vi "映射处理_kc705.vi"() -> ()   [LabVIEW 2017]
uses:
  <vilib>/Utility/file.llb/Read Delimited Spreadsheet (string).vi
panel:
  in  "-N":bool=TRUE
  in  "prefix":string="HPC_"
  out "initialized array":string[][](array[string])
  out "all rows":string[][](array[string])=[["VO0", "LA02_P"], ["VO1", "HA06_P"], ["VO2", "HA10_P"], ["VO3", "HA15_P"], ["VO4", "LA20_P"], ["VO5", "HB02_P"], ["VO6", "HB00_P"], ["VO7", "LA24_P"], ["VO8", "HB13_P"], ["VO9", "HB16_P"], ["VO10", "LA01_P"], ["VO11", "HA08_P"], ["VO12", "HA12_P"], ["VO13", "HA20_P"], ["VO14", "LA19_P"], ["VO15", "LA23_P"], ["VO16", "HB04_P"], ["VO17", "HB08_P"], ["VO18", "HB15_P"], ["VO19", "HB21_P"], ["VO20", "HA09_P"], ["VO21", "HA13_P"], ["VO22", "HA16_P"], ["VO23", "LA15_P"], ["VO24", "HA23_P"], ["VO25", "LA21_P"], ["VO26", "HB09_P"], ["VO27", "HB11_P"], ["VO28", "HB12_P"], ["VO29", "HB14_P"], ["VO30", "HA07_P"], ["VO31", "LA05_P"], ["VO32", "LA10_P"], ["VO33", "HA17_P"], ["VO34", "HA22_P"], ["VO35", "HB01_P"], ["VO36", "HB07_P"], ["VO37", "HB06_P"], ["VO38", "LA31_P"], ["VO39", "HB18_P"], ["VO40", "LA03_P"], ["VO41", "LA08_P"], ["VO42", "HA14_P"], ["VO43", "HA18_P"], ["VO45", "HB05_P"], ["VO46", "LA25_P"], ["VO47", "LA28_P"], ["VO48", "HB19_P"], ["VO49", "LA32_P"], ["VO50", "LA04_P"], ["VO51", "HA11_P"], ["VO52", "LA09_P"], ["VO53", "HA19_P"], ["VO54", "LA18_P"], ["VO55", "LA27_P"], ["VO56", "LA26_P"], ["VO57", "LA29_P"], ["VO58", "LA30_P"], ["VO59", "HB17_P"], ["VO60", "LA06_P"], ["VO61", "LA07_P"], ["VO62", "LA12_P"], ["VO63", "HA21_P"]]
  out "subarray 2":string[](array[string])=["LA02_P", "HA06_P", "HA10_P", "HA15_P", "LA20_P", "HB02_P", "HB00_P", "LA24_P", "HB13_P", "HB16_P", "LA01_P", "HA08_P", "HA12_P", "HA20_P", "LA19_P", "LA23_P", "HB04_P", "HB08_P", "HB15_P", "HB21_P", "HA09_P", "HA13_P", "HA16_P", "LA15_P", "HA23_P", "LA21_P", "HB09_P", "HB11_P", "HB12_P", "HB14_P", "HA07_P", "LA05_P", "LA10_P", "HA17_P", "HA22_P", "HB01_P", "HB07_P", "HB06_P", "LA31_P", "HB18_P", "LA03_P", "LA08_P", "HA14_P", "HA18_P", "HB05_P", "LA25_P", "LA28_P", "HB19_P", "LA32_P", "LA04_P", "HA11_P", "LA09_P", "HA19_P", "LA18_P", "LA27_P", "LA26_P", "LA29_P", "LA30_P", "HB17_P", "LA06_P", "LA07_P", "LA12_P", "HA21_P"]
  out "subarray":string[](array[string])=["set_property PACKAGE_PIN Y20 [get_ports SFP_TX_DISABLE]", "set_property IOSTANDARD LVCMOS25 [get_ports SFP_TX_DISABLE]", "set_property PACKAGE_PIN Y23 [get_ports USER_SMA_GPIO_P]", "set_property IOSTANDARD LVCMOS25 [get_ports USER_SMA_GPIO_P]", "set_property PACKAGE_PIN Y24 [get_ports USER_SMA_GPIO_N]", "set_property IOSTANDARD LVCMOS25 [get_ports USER_SMA_GPIO_N]", "set_property PACKAGE_PIN Y21 [get_ports SDIO_SDWP]", "set_property IOSTANDARD LVCMOS25 [get_ports SDIO_SDWP]", "set_property PACKAGE_PIN AA21 [get_ports SDIO_SDDET]", "set_property IOSTANDARD LVCMOS25 [get_ports SDIO_SDDET]", "set_property PACKAGE_PIN AB22 [get_ports SDIO_CMD_LS]", "set_property IOSTANDARD LVCMOS25 [get_ports SDIO_CMD_LS]", "set_property PACKAGE_PIN AB23 [get_ports SDIO_CLK_LS]", "set_property IOSTANDARD LVCMOS25 [get_ports SDIO_CLK_LS]", "set_property PACKAGE_PIN AA22 [get_ports SDIO_DAT2_LS]", "set_property IOSTANDARD LVCMOS25 [get_ports SDIO_DAT2_LS]", "set_property PACKAGE_PIN AA23 [get_ports SDIO_DAT1_LS]", "set_property IOSTANDARD LVCMOS25 [get_ports SDIO_DAT1_LS]", "set_property PACKAGE_PIN AC20 [get_ports SDIO_DAT0_LS]", "set_property IOSTANDARD LVCMOS25 [get_ports SDIO_DAT0_LS]", "set_property PACKAGE_PIN AC21 [get_ports SDIO_CD_DAT3_LS]", "set_property IOSTANDARD LVCMOS25 [get_ports SDIO_CD_DAT3_LS]", "set_property PACKAGE_PIN AA20 [get_ports FMC_LPC_LA12_P]", "set_property IOSTANDARD LVCMOS25 [get_ports FMC_LPC_LA12_P]", "set_property PACKAGE_PIN AB20 [get_ports FMC_LPC_LA12_N]", "set_property IOSTANDARD LVCMOS25 [get_ports FMC_LPC_LA12_N]", "set_property PACKAGE_PIN AB24 [get_ports FMC_LPC_LA13_P]", "set_property IOSTANDARD LVCMOS25 [get_ports FMC_LPC_LA13_P]", "set_property PACKAGE_PIN AC25 [get_ports FMC_LPC_LA13_N]", "set_property IOSTANDARD LVCMOS25 [get_ports FMC_LPC_LA13_N]", "set_property PACKAGE_PIN AC22 [get_ports FMC_LPC_LA16_P]", "set_property IOSTANDARD LVCMOS25 [get_ports FMC_LPC_LA16_P]", "set_property PACKAGE_PIN AD22 [get_ports FMC_LPC_LA16_N]", "set_property IOSTANDARD LVCMOS25 [get_ports FMC_LPC_LA16_N]", "set_property PACKAGE_PIN AC24 [get_ports FMC_LPC_LA15_P]", "set_property IOSTANDARD LVCMOS25 [get_ports FMC_LPC_LA15_P]", "set_property PACKAGE_PIN AD24 [get_ports FMC_LPC_LA15_N]", "set_property IOSTANDARD LVCMOS25 [get_ports FMC_LPC_LA15_N]", "set_property PACKAGE_PIN AD21 [get_ports FMC_LPC_LA14_P]", "set_property IOSTANDARD LVCMOS25 [get_ports FMC_LPC_LA14_P]", "set_property PACKAGE_PIN AE21 [get_ports FMC_LPC_LA14_N]", "set_property IOSTANDARD LVCMOS25 [get_ports FMC_LPC_LA14_N]", "set_property PACKAGE_PIN AE23 [get_ports FMC_LPC_LA01_CC_P]", "set_property IOSTANDARD LVCMOS25 [get_ports FMC_LPC_LA01_CC_P]", "set_property PACKAGE_PIN AF23 [get_ports FMC_LPC_LA01_CC_N]", "set_property IOSTANDARD LVCMOS25 [get_ports FMC_LPC_LA01_CC_N]", "set_property PACKAGE_PIN AD23 [get_ports FMC_LPC_LA00_CC_P]", "set_property IOSTANDARD LVCMOS25 [get_ports FMC_LPC_LA00_CC_P]", "set_property PACKAGE_PIN AE24 [get_ports FMC_LPC_LA00_CC_N]", "set_property IOSTANDARD LVCMOS25 [get_ports FMC_LPC_LA00_CC_N]", "set_property PACKAGE_PIN AF22 [get_ports FMC_LPC_CLK0_M2C_P]", "set_property IOSTANDARD LVCMOS25 [get_ports FMC_LPC_CLK0_M2C_P]", "set_property PACKAGE_PIN AG23 [get_ports FMC_LPC_CLK0_M2C_N]", "set_property IOSTANDARD LVCMOS25 [get_ports FMC_LPC_CLK0_M2C_N]", "set_property PACKAGE_PIN AG24 [get_ports SI5326_INT_ALM_LS]", "set_property IOSTANDARD LVCMOS25 [get_ports SI5326_INT_ALM_LS]", "set_property PACKAGE_PIN AH24 [get_ports HDMI_INT]", "set_property IOSTANDARD LVCMOS25 [get_ports HDMI_INT]", "set_property PACKAGE_PIN AJ24 [get_ports FMC_LPC_LA10_P]", "set_property IOSTANDARD LVCMOS25 [get_ports FMC_LPC_LA10_P]", "set_property PACKAGE_PIN AK25 [get_ports FMC_LPC_LA10_N]", "set_property IOSTANDARD LVCMOS25 [get_ports FMC_LPC_LA10_N]", "set_property PACKAGE_PIN AE25 [get_ports FMC_LPC_LA11_P]", "set_property IOSTANDARD LVCMOS25 [get_ports FMC_LPC_LA11_P]", "set_property PACKAGE_PIN AF25 [get_ports FMC_LPC_LA11_N]", "set_property IOSTANDARD LVCMOS25 [get_ports FMC_LPC_LA11_N]", "set_property PACKAGE_PIN AK23 [get_ports FMC_LPC_LA09_P]", "set_property IOSTANDARD LVCMOS25 [get_ports FMC_LPC_LA09_P]", "set_property PACKAGE_PIN AK24 [get_ports FMC_LPC_LA09_N]", "set_property IOSTANDARD LVCMOS25 [get_ports FMC_LPC_LA09_N]", "set_property PACKAGE_PIN AG25 [get_ports FMC_LPC_LA07_P]", "set_property IOSTANDARD LVCMOS25 [get_ports FMC_LPC_LA07_P]", "set_property PACKAGE_PIN AH25 [get_ports FMC_LPC_LA07_N]", "set_property IOSTANDARD LVCMOS25 [get_ports FMC_LPC_LA07_N]", "set_property PACKAGE_PIN AF20 [get_ports FMC_LPC_LA02_P]", "set_property IOSTANDARD LVCMOS25 [get_ports FMC_LPC_LA02_P]", "set_property PACKAGE_PIN AF21 [get_ports FMC_LPC_LA02_N]", "set_property IOSTANDARD LVCMOS25 [get_ports FMC_LPC_LA02_N]", "set_property PACKAGE_PIN AG22 [get_ports FMC_LPC_LA05_P]", "set_property IOSTANDARD LVCMOS25 [get_ports FMC_LPC_LA05_P]", "set_property PACKAGE_PIN AH22 [get_ports FMC_LPC_LA05_N]", "set_property IOSTANDARD LVCMOS25 [get_ports FMC_LPC_LA05_N]", "set_property PACKAGE_PIN AJ22 [get_ports FMC_LPC_LA08_P]", "set_property IOSTANDARD LVCMOS25 [get_ports FMC_LPC_LA08_P]", "set_property PACKAGE_PIN AJ23 [get_ports FMC_LPC_LA08_N]", "set_property IOSTANDARD LVCMOS25 [get_ports FMC_LPC_LA08_N]", "set_property PACKAGE_PIN AG20 [get_ports FMC_LPC_LA03_P]", "set_property IOSTANDARD LVCMOS25 [get_ports FMC_LPC_LA03_P]", "set_property PACKAGE_PIN AH20 [get_ports FMC_LPC_LA03_N]", "set_property IOSTANDARD LVCMOS25 [get_ports FMC_LPC_LA03_N]", "set_property PACKAGE_PIN AH21 [get_ports FMC_LPC_LA04_P]", "set_property IOSTANDARD LVCMOS25 [get_ports FMC_LPC_LA04_P]", "set_property PACKAGE_PIN AJ21 [get_ports FMC_LPC_LA04_N]", "set_property IOSTANDARD LVCMOS25 [get_ports FMC_LPC_LA04_N]", "set_property PACKAGE_PIN AK20 [get_ports FMC_LPC_LA06_P]", "set_property IOSTANDARD LVCMOS25 [get_ports FMC_LPC_LA06_P]", "set_property PACKAGE_PIN AK21 [get_ports FMC_LPC_LA06_N]", "set_property IOSTANDARD LVCMOS25 [get_ports FMC_LPC_LA06_N]", "set_property PACKAGE_PIN AE20 [get_ports SI5326_RST_LS]", "set_property IOSTANDARD LVCMOS25 [get_ports SI5326_RST_LS]", "set_property PACKAGE_PIN Y25 [get_ports ROTARY_INCB]", "set_property IOSTANDARD LVCMOS25 [get_ports ROTARY_INCB]", "set_property PACKAGE_PIN Y26 [get_ports ROTARY_INCA]", "set_property IOSTANDARD LVCMOS25 [get_ports ROTARY_INCA]", "set_property PACKAGE_PIN AA26 [get_ports ROTARY_PUSH]", "set_property IOSTANDARD LVCMOS25 [get_ports ROTARY_PUSH]", "set_property PACKAGE_PIN W27 [get_ports REC_CLOCK_C_P]", "set_property IOSTANDARD LVDS_25 [get_ports REC_CLOCK_C_P]", "set_property PACKAGE_PIN W28 [get_ports REC_CLOCK_C_N]", "set_property IOSTANDARD LVDS_25 [get_ports REC_CLOCK_C_N]", "set_property PACKAGE_PIN Y28 [get_ports GPIO_DIP_SW3]", "set_property IOSTANDARD LVCMOS25 [get_ports GPIO_DIP_SW3]", "set_property PACKAGE_PIN AA28 [get_ports GPIO_DIP_SW2]", "set_property IOSTANDARD LVCMOS25 [get_ports GPIO_DIP_SW2]", "set_property PACKAGE_PIN W29 [get_ports GPIO_DIP_SW1]", "set_property IOSTANDARD LVCMOS25 [get_ports GPIO_DIP_SW1]", "set_property PACKAGE_PIN Y29 [get_ports GPIO_DIP_SW0]", "set_property IOSTANDARD LVCMOS25 [get_ports GPIO_DIP_SW0]", "set_property PACKAGE_PIN AA27 [get_ports XADC_GPIO_3]", "set_property IOSTANDARD LVCMOS25 [get_ports XADC_GPIO_3]", "set_property PACKAGE_PIN AB28 [get_ports XADC_GPIO_2]", "set_property IOSTANDARD LVCMOS25 [get_ports XADC_GPIO_2]", "set_property PACKAGE_PIN AA25 [get_ports XADC_GPIO_1]", "set_property IOSTANDARD LVCMOS25 [get_ports XADC_GPIO_1]", "set_property PACKAGE_PIN AB25 [get_ports XADC_GPIO_0]", "set_property IOSTANDARD LVCMOS25 [get_ports XADC_GPIO_0]", "set_property PACKAGE_PIN AC29 [get_ports FMC_LPC_LA33_P]", "set_property IOSTANDARD LVCMOS25 [get_ports FMC_LPC_LA33_P]", "set_property PACKAGE_PIN AC30 [get_ports FMC_LPC_LA33_N]", "set_property IOSTANDARD LVCMOS25 [get_ports FMC_LPC_LA33_N]", "set_property PACKAGE_PIN Y30 [get_ports FMC_LPC_LA32_P]", "set_property IOSTANDARD LVCMOS25 [get_ports FMC_LPC_LA32_P]", "set_property PACKAGE_PIN AA30 [get_ports FMC_LPC_LA32_N]", "set_property IOSTANDARD LVCMOS25 [get_ports FMC_LPC_LA32_N]", "set_property PACKAGE_PIN AD29 [get_ports FMC_LPC_LA31_P]", "set_property IOSTANDARD LVCMOS25 [get_ports FMC_LPC_LA31_P]", "set_property PACKAGE_PIN AE29 [get_ports FMC_LPC_LA31_N]", "set_property IOSTANDARD LVCMOS25 [get_ports FMC_LPC_LA31_N]", "set_property PACKAGE_PIN AB29 [get_ports FMC_LPC_LA30_P]", "set_property IOSTANDARD LVCMOS25 [get_ports FMC_LPC_LA30_P]", "set_property PACKAGE_PIN AB30 [get_ports FMC_LPC_LA30_N]", "set_property IOSTANDARD LVCMOS25 [get_ports FMC_LPC_LA30_N]", "set_property PACKAGE_PIN AD27 [get_ports FMC_LPC_LA18_CC_P]", "set_property IOSTANDARD LVCMOS25 [get_ports FMC_LPC_LA18_CC_P]", "set_property PACKAGE_PIN AD28 [get_ports FMC_LPC_LA18_CC_N]", "set_property IOSTANDARD LVCMOS25 [get_ports FMC_LPC_LA18_CC_N]", "set_property PACKAGE_PIN AB27 [get_ports FMC_LPC_LA17_CC_P]", "set_property IOSTANDARD LVCMOS25 [get_ports FMC_LPC_LA17_CC_P]", "set_property PACKAGE_PIN AC27 [get_ports FMC_LPC_LA17_CC_N]", "set_property IOSTANDARD LVCMOS25 [get_ports FMC_LPC_LA17_CC_N]", "set_property PACKAGE_PIN AG29 [get_ports FMC_LPC_CLK1_M2C_P]", "set_property IOSTANDARD LVCMOS25 [get_ports FMC_LPC_CLK1_M2C_P]", "set_property PACKAGE_PIN AH29 [get_ports FMC_LPC_CLK1_M2C_N]", "set_property IOSTANDARD LVCMOS25 [get_ports FMC_LPC_CLK1_M2C_N]", "set_property PACKAGE_PIN AE28 [get_ports FMC_LPC_LA29_P]", "set_property IOSTANDARD LVCMOS25 [get_ports FMC_LPC_LA29_P]", "set_property PACKAGE_PIN AF28 [get_ports FMC_LPC_LA29_N]", "set_property IOSTANDARD LVCMOS25 [get_ports FMC_LPC_LA29_N]", "set_property PACKAGE_PIN AK29 [get_ports FMC_LPC_LA26_P]", "set_property IOSTANDARD LVCMOS25 [get_ports FMC_LPC_LA26_P]", "set_property PACKAGE_PIN AK30 [get_ports FMC_LPC_LA26_N]", "set_property IOSTANDARD LVCMOS25 [get_ports FMC_LPC_LA26_N]", "set_property PACKAGE_PIN AE30 [get_ports FMC_LPC_LA28_P]", "set_property IOSTANDARD LVCMOS25 [get_ports FMC_LPC_LA28_P]", "set_property PACKAGE_PIN AF30 [get_ports FMC_LPC_LA28_N]", "set_property IOSTANDARD LVCMOS25 [get_ports FMC_LPC_LA28_N]", "set_property PACKAGE_PIN AJ28 [get_ports FMC_LPC_LA27_P]", "set_property IOSTANDARD LVCMOS25 [get_ports FMC_LPC_LA27_P]", "set_property PACKAGE_PIN AJ29 [get_ports FMC_LPC_LA27_N]", "set_property IOSTANDARD LVCMOS25 [get_ports FMC_LPC_LA27_N]", "set_property PACKAGE_PIN AG30 [get_ports FMC_LPC_LA24_P]", "set_property IOSTANDARD LVCMOS25 [get_ports FMC_LPC_LA24_P]", "set_property PACKAGE_PIN AH30 [get_ports FMC_LPC_LA24_N]", "set_property IOSTANDARD LVCMOS25 [get_ports FMC_LPC_LA24_N]", "set_property PACKAGE_PIN AC26 [get_ports FMC_LPC_LA25_P]", "set_property IOSTANDARD LVCMOS25 [get_ports FMC_LPC_LA25_P]", "set_property PACKAGE_PIN AD26 [get_ports FMC_LPC_LA25_N]", "set_property IOSTANDARD LVCMOS25 [get_ports FMC_LPC_LA25_N]", "set_property PACKAGE_PIN AJ27 [get_ports FMC_LPC_LA22_P]", "set_property IOSTANDARD LVCMOS25 [get_ports FMC_LPC_LA22_P]", "set_property PACKAGE_PIN AK28 [get_ports FMC_LPC_LA22_N]", "set_property IOSTANDARD LVCMOS25 [get_ports FMC_LPC_LA22_N]", "set_property PACKAGE_PIN AG27 [get_ports FMC_LPC_LA21_P]", "set_property IOSTANDARD LVCMOS25 [get_ports FMC_LPC_LA21_P]", "set_property PACKAGE_PIN AG28 [get_ports FMC_LPC_LA21_N]", "set_property IOSTANDARD LVCMOS25 [get_ports FMC_LPC_LA21_N]", "set_property PACKAGE_PIN AH26 [get_ports FMC_LPC_LA23_P]", "set_property IOSTANDARD LVCMOS25 [get_ports FMC_LPC_LA23_P]", "set_property PACKAGE_PIN AH27 [get_ports FMC_LPC_LA23_N]", "set_property IOSTANDARD LVCMOS25 [get_ports FMC_LPC_LA23_N]", "set_property PACKAGE_PIN AF26 [get_ports FMC_LPC_LA20_P]", "set_property IOSTANDARD LVCMOS25 [get_ports FMC_LPC_LA20_P]", "set_property PACKAGE_PIN AF27 [get_ports FMC_LPC_LA20_N]", "set_property IOSTANDARD LVCMOS25 [get_ports FMC_LPC_LA20_N]", "set_property PACKAGE_PIN AJ26 [get_ports FMC_LPC_LA19_P]", "set_property IOSTANDARD LVCMOS25 [get_ports FMC_LPC_LA19_P]", "set_property PACKAGE_PIN AK26 [get_ports FMC_LPC_LA19_N]", "set_property IOSTANDARD LVCMOS25 [get_ports FMC_LPC_LA19_N]", "set_property PACKAGE_PIN AE26 [get_ports GPIO_LED_4_LS]", "set_property IOSTANDARD LVCMOS25 [get_ports GPIO_LED_4_LS]", "set_property PACKAGE_PIN R19 [get_ports PHY_RXD4]", "set_property IOSTANDARD LVCMOS25 [get_ports PHY_RXD4]", "set_property PACKAGE_PIN P24 [get_ports FLASH_D0]", "set_property IOSTANDARD LVCMOS25 [get_ports FLASH_D0]", "set_property PACKAGE_PIN R25 [get_ports FLASH_D1]", "set_property IOSTANDARD LVCMOS25 [get_ports FLASH_D1]", "set_property PACKAGE_PIN R20 [get_ports FLASH_D2]", "set_property IOSTANDARD LVCMOS25 [get_ports FLASH_D2]", "set_property PACKAGE_PIN R21 [get_ports FLASH_D3]", "set_property IOSTANDARD LVCMOS25 [get_ports FLASH_D3]", "set_property PACKAGE_PIN R23 [get_ports PHY_MDC]", "set_property IOSTANDARD LVCMOS25 [get_ports PHY_MDC]", "set_property PACKAGE_PIN R24 [get_ports FPGA_EMCCLK]", "set_property IOSTANDARD LVCMOS25 [get_ports FPGA_EMCCLK]", "set_property PACKAGE_PIN T20 [get_ports FLASH_D4]", "set_property IOSTANDARD LVCMOS25 [get_ports FLASH_D4]", "set_property PACKAGE_PIN T21 [get_ports FLASH_D5]", "set_property IOSTANDARD LVCMOS25 [get_ports FLASH_D5]", "set_property PACKAGE_PIN T22 [get_ports FLASH_D6]", "set_property IOSTANDARD LVCMOS25 [get_ports FLASH_D6]", "set_property PACKAGE_PIN T23 [get_ports FLASH_D7]", "set_property IOSTANDARD LVCMOS25 [get_ports FLASH_D7]", "set_property PACKAGE_PIN U19 [get_ports FPGA_FCS]", "set_property IOSTANDARD LVCMOS25 [get_ports FPGA_FCS]", "set_property PACKAGE_PIN U20 [get_ports FLASH_D8]", "set_property IOSTANDARD LVCMOS25 [get_ports FLASH_D8]", "set_property PACKAGE_PIN P29 [get_ports FLASH_D9]", "set_property IOSTANDARD LVCMOS25 [get_ports FLASH_D9]", "set_property PACKAGE_PIN R29 [get_ports FLASH_D10]", "set_property IOSTANDARD LVCMOS25 [get_ports FLASH_D10]", "set_property PACKAGE_PIN P27 [get_ports FLASH_D11]", "set_property IOSTANDARD LVCMOS25 [get_ports FLASH_D11]", "set_property PACKAGE_PIN P28 [get_ports FLASH_D12]", "set_property IOSTANDARD LVCMOS25 [get_ports FLASH_D12]", "set_property PACKAGE_PIN R30 [get_ports PHY_CRS]", "set_property IOSTANDARD LVCMOS25 [get_ports PHY_CRS]", "set_property PACKAGE_PIN T30 [get_ports FLASH_D13]", "set_property IOSTANDARD LVCMOS25 [get_ports FLASH_D13]", "set_property PACKAGE_PIN P26 [get_ports FLASH_D14]", "set_property IOSTANDARD LVCMOS25 [get_ports FLASH_D14]", "set_property PACKAGE_PIN R26 [get_ports FLASH_D15]", "set_property IOSTANDARD LVCMOS25 [get_ports FLASH_D15]", "set_property PACKAGE_PIN R28 [get_ports PHY_RXCTL_RXDV]", "set_property IOSTANDARD LVCMOS25 [get_ports PHY_RXCTL_RXDV]", "set_property PACKAGE_PIN T28 [get_ports PHY_RXD7]", "set_property IOSTANDARD LVCMOS25 [get_ports PHY_RXD7]", "set_property PACKAGE_PIN T26 [get_ports PHY_RXD6]", "set_property IOSTANDARD LVCMOS25 [get_ports PHY_RXD6]", "set_property PACKAGE_PIN T27 [get_ports PHY_RXD5]", "set_property IOSTANDARD LVCMOS25 [get_ports PHY_RXD5]", "set_property PACKAGE_PIN U27 [get_ports PHY_RXCLK]", "set_property IOSTANDARD LVCMOS25 [get_ports PHY_RXCLK]", "set_property PACKAGE_PIN U28 [get_ports PHY_RXD3]", "set_property IOSTANDARD LVCMOS25 [get_ports PHY_RXD3]", "set_property PACKAGE_PIN T25 [get_ports PHY_RXD2]", "set_property IOSTANDARD LVCMOS25 [get_ports PHY_RXD2]", "set_property PACKAGE_PIN U25 [get_ports PHY_RXD1]", "set_property IOSTANDARD LVCMOS25 [get_ports PHY_RXD1]", "set_property PACKAGE_PIN U29 [get_ports FLASH_WAIT]", "set_property IOSTANDARD LVCMOS25 [get_ports FLASH_WAIT]", "set_property PACKAGE_PIN U30 [get_ports PHY_RXD0]", "set_property IOSTANDARD LVCMOS25 [get_ports PHY_RXD0]", "set_property PACKAGE_PIN V26 [get_ports PHY_RXER]", "set_property IOSTANDARD LVCMOS25 [get_ports PHY_RXER]", "set_property PACKAGE_PIN V27 [get_ports FLASH_A15]", "set_property IOSTANDARD LVCMOS25 [get_ports FLASH_A15]", "set_property PACKAGE_PIN V29 [get_ports FLASH_A14]", "set_property IOSTANDARD LVCMOS25 [get_ports FLASH_A14]", "set_property PACKAGE_PIN V30 [get_ports FLASH_A13]", "set_property IOSTANDARD LVCMOS25 [get_ports FLASH_A13]", "set_property PACKAGE_PIN V25 [get_ports FLASH_A12]", "set_property IOSTANDARD LVCMOS25 [get_ports FLASH_A12]", "set_property PACKAGE_PIN W26 [get_ports FLASH_A11]", "set_property IOSTANDARD LVCMOS25 [get_ports FLASH_A11]", "set_property PACKAGE_PIN V19 [get_ports FLASH_A10]", "set_property IOSTANDARD LVCMOS25 [get_ports FLASH_A10]", "set_property PACKAGE_PIN V20 [get_ports FLASH_A9]", "set_property IOSTANDARD LVCMOS25 [get_ports FLASH_A9]", "set_property PACKAGE_PIN W23 [get_ports FLASH_A8]", "set_property IOSTANDARD LVCMOS25 [get_ports FLASH_A8]", "set_property PACKAGE_PIN W24 [get_ports FLASH_A7]", "set_property IOSTANDARD LVCMOS25 [get_ports FLASH_A7]", "set_property PACKAGE_PIN U22 [get_ports SM_FAN_TACH]", "set_property IOSTANDARD LVCMOS25 [get_ports SM_FAN_TACH]", "set_property PACKAGE_PIN U23 [get_ports FLASH_A6]", "set_property IOSTANDARD LVCMOS25 [get_ports FLASH_A6]", "set_property PACKAGE_PIN V21 [get_ports FLASH_A5]", "set_property IOSTANDARD LVCMOS25 [get_ports FLASH_A5]", "set_property PACKAGE_PIN V22 [get_ports FLASH_A4]", "set_property IOSTANDARD LVCMOS25 [get_ports FLASH_A4]", "set_property PACKAGE_PIN U24 [get_ports FLASH_A3]", "set_property IOSTANDARD LVCMOS25 [get_ports FLASH_A3]", "set_property PACKAGE_PIN V24 [get_ports FLASH_A2]", "set_property IOSTANDARD LVCMOS25 [get_ports FLASH_A2]", "set_property PACKAGE_PIN W21 [get_ports FLASH_A1]", "set_property IOSTANDARD LVCMOS25 [get_ports FLASH_A1]", "set_property PACKAGE_PIN W22 [get_ports FLASH_A0]", "set_property IOSTANDARD LVCMOS25 [get_ports FLASH_A0]", "set_property PACKAGE_PIN W19 [get_ports PHY_COL]", "set_property IOSTANDARD LVCMOS25 [get_ports PHY_COL]", "set_property PACKAGE_PIN M19 [get_ports USB_TX]", "set_property IOSTANDARD LVCMOS25 [get_ports USB_TX]", "set_property PACKAGE_PIN J23 [get_ports XADC_VAUX0P_R]", "set_property IOSTANDARD LVCMOS25 [get_ports XADC_VAUX0P_R]", "set_property PACKAGE_PIN J24 [get_ports XADC_VAUX0N_R]", "set_property IOSTANDARD LVCMOS25 [get_ports XADC_VAUX0N_R]", "set_property PACKAGE_PIN L22 [get_ports XADC_VAUX8P_R]", "set_property IOSTANDARD LVCMOS25 [get_ports XADC_VAUX8P_R]", "set_property PACKAGE_PIN L23 [get_ports XADC_VAUX8N_R]", "set_property IOSTANDARD LVCMOS25 [get_ports XADC_VAUX8N_R]", "set_property PACKAGE_PIN K23 [get_ports USB_RTS]", "set_property IOSTANDARD LVCMOS25 [get_ports USB_RTS]", "set_property PACKAGE_PIN K24 [get_ports USB_RX]", "set_property IOSTANDARD LVCMOS25 [get_ports USB_RX]", "set_property PACKAGE_PIN L21 [get_ports IIC_SDA_MAIN]", "set_property IOSTANDARD LVCMOS25 [get_ports IIC_SDA_MAIN]", "set_property PACKAGE_PIN K21 [get_ports IIC_SCL_MAIN]", "set_property IOSTANDARD LVCMOS25 [get_ports IIC_SCL_MAIN]", "set_property PACKAGE_PIN J21 [get_ports PHY_MDIO]", "set_property IOSTANDARD LVCMOS25 [get_ports PHY_MDIO]", "set_property PACKAGE_PIN J22 [get_ports FMC_LPC_PRSNT_M2C_B_LS]", "set_property IOSTANDARD LVCMOS25 [get_ports FMC_LPC_PRSNT_M2C_B_LS]", "set_property PACKAGE_PIN M20 [get_ports FMC_HPC_PRSNT_M2C_B_LS]", "set_property IOSTANDARD LVCMOS25 [get_ports FMC_HPC_PRSNT_M2C_B_LS]", "set_property PACKAGE_PIN L20 [get_ports PHY_RESET]", "set_property IOSTANDARD LVCMOS25 [get_ports PHY_RESET]", "set_property PACKAGE_PIN J29 [get_ports FMC_HPC_PG_M2C_LS]", "set_property IOSTANDARD LVCMOS25 [get_ports FMC_HPC_PG_M2C_LS]", "set_property PACKAGE_PIN H29 [get_ports FMC_C2M_PG_LS]", "set_property IOSTANDARD LVCMOS25 [get_ports FMC_C2M_PG_LS]", "set_property PACKAGE_PIN J27 [get_ports FMC_VADJ_ON_B_LS]", "set_property IOSTANDARD LVCMOS25 [get_ports FMC_VADJ_ON_B_LS]", "set_property PACKAGE_PIN J28 [get_ports PHY_TXD7]", "set_property IOSTANDARD LVCMOS25 [get_ports PHY_TXD7]", "set_property PACKAGE_PIN L30 [get_ports PHY_TXD6]", "set_property IOSTANDARD LVCMOS25 [get_ports PHY_TXD6]", "set_property PACKAGE_PIN K30 [get_ports PHY_TXC_GTXCLK]", "set_property IOSTANDARD LVCMOS25 [get_ports PHY_TXC_GTXCLK]", "set_property PACKAGE_PIN K26 [get_ports PHY_TXD5]", "set_property IOSTANDARD LVCMOS25 [get_ports PHY_TXD5]", "set_property PACKAGE_PIN J26 [get_ports PHY_TXD4]", "set_property IOSTANDARD LVCMOS25 [get_ports PHY_TXD4]", "set_property PACKAGE_PIN L26 [get_ports SM_FAN_PWM]", "set_property IOSTANDARD LVCMOS25 [get_ports SM_FAN_PWM]", "set_property PACKAGE_PIN L27 [get_ports USB_CTS]", "set_property IOSTANDARD LVCMOS25 [get_ports USB_CTS]", "set_property PACKAGE_PIN L25 [get_ports USER_SMA_CLOCK_P]", "set_property IOSTANDARD LVDS_25 [get_ports USER_SMA_CLOCK_P]", "set_property PACKAGE_PIN K25 [get_ports USER_SMA_CLOCK_N]", "set_property IOSTANDARD LVDS_25 [get_ports USER_SMA_CLOCK_N]", "set_property PACKAGE_PIN K28 [get_ports USER_CLOCK_P]", "set_property IOSTANDARD LVDS_25 [get_ports USER_CLOCK_P]", "set_property PACKAGE_PIN K29 [get_ports USER_CLOCK_N]", "set_property IOSTANDARD LVDS_25 [get_ports USER_CLOCK_N]", "set_property PACKAGE_PIN M28 [get_ports PHY_TXCLK]", "set_property IOSTANDARD LVCMOS25 [get_ports PHY_TXCLK]", "set_property PACKAGE_PIN L28 [get_ports PHY_TXD3]", "set_property IOSTANDARD LVCMOS25 [get_ports PHY_TXD3]", "set_property PACKAGE_PIN M29 [get_ports PHY_TXD2]", "set_property IOSTANDARD LVCMOS25 [get_ports PHY_TXD2]", "set_property PACKAGE_PIN M30 [get_ports FLASH_ADV_B]", "set_property IOSTANDARD LVCMOS25 [get_ports FLASH_ADV_B]", "set_property PACKAGE_PIN N27 [get_ports PHY_TXD0]", "set_property IOSTANDARD LVCMOS25 [get_ports PHY_TXD0]", "set_property PACKAGE_PIN M27 [get_ports PHY_TXCTL_TXEN]", "set_property IOSTANDARD LVCMOS25 [get_ports PHY_TXCTL_TXEN]", "set_property PACKAGE_PIN N29 [get_ports PHY_TXER]", "set_property IOSTANDARD LVCMOS25 [get_ports PHY_TXER]", "set_property PACKAGE_PIN N30 [get_ports PHY_INT]", "set_property IOSTANDARD LVCMOS25 [get_ports PHY_INT]", "set_property PACKAGE_PIN N25 [get_ports PHY_TXD1]", "set_property IOSTANDARD LVCMOS25 [get_ports PHY_TXD1]", "set_property PACKAGE_PIN N26 [get_ports FLASH_A23]", "set_property IOSTANDARD LVCMOS25 [get_ports FLASH_A23]", "set_property PACKAGE_PIN N19 [get_ports FLASH_A22]", "set_property IOSTANDARD LVCMOS25 [get_ports FLASH_A22]", "set_property PACKAGE_PIN N20 [get_ports FLASH_A21]", "set_property IOSTANDARD LVCMOS25 [get_ports FLASH_A21]", "set_property PACKAGE_PIN N21 [get_ports FLASH_A20]", "set_property IOSTANDARD LVCMOS25 [get_ports FLASH_A20]", "set_property PACKAGE_PIN N22 [get_ports FLASH_A19]", "set_property IOSTANDARD LVCMOS25 [get_ports FLASH_A19]", "set_property PACKAGE_PIN P23 [get_ports IIC_MUX_RESET_B]", "set_property IOSTANDARD LVCMOS25 [get_ports IIC_MUX_RESET_B]", "set_property PACKAGE_PIN N24 [get_ports FLASH_A18]", "set_property IOSTANDARD LVCMOS25 [get_ports FLASH_A18]", "set_property PACKAGE_PIN P21 [get_ports FLASH_A17]", "set_property IOSTANDARD LVCMOS25 [get_ports FLASH_A17]", "set_property PACKAGE_PIN P22 [get_ports FLASH_A16]", "set_property IOSTANDARD LVCMOS25 [get_ports FLASH_A16]", "set_property PACKAGE_PIN M24 [get_ports FLASH_OE_B]", "set_property IOSTANDARD LVCMOS25 [get_ports FLASH_OE_B]", "set_property PACKAGE_PIN M25 [get_ports FLASH_FWE_B]", "set_property IOSTANDARD LVCMOS25 [get_ports FLASH_FWE_B]", "set_property PACKAGE_PIN M22 [get_ports FLASH_A25]", "set_property IOSTANDARD LVCMOS25 [get_ports FLASH_A25]", "set_property PACKAGE_PIN M23 [get_ports FLASH_A24]", "set_property IOSTANDARD LVCMOS25 [get_ports FLASH_A24]", "set_property PACKAGE_PIN P19 [get_ports SFP_LOS_LS]", "set_property IOSTANDARD LVCMOS25 [get_ports SFP_LOS_LS]", "set_property PACKAGE_PIN F23 [get_ports PCIE_WAKE_B_LS]", "set_property IOSTANDARD LVCMOS25 [get_ports PCIE_WAKE_B_LS]", "set_property PACKAGE_PIN B23 [get_ports HDMI_R_D0]", "set_property IOSTANDARD LVCMOS25 [get_ports HDMI_R_D0]", "set_property PACKAGE_PIN A23 [get_ports HDMI_R_D1]", "set_property IOSTANDARD LVCMOS25 [get_ports HDMI_R_D1]", "set_property PACKAGE_PIN E23 [get_ports HDMI_R_D2]", "set_property IOSTANDARD LVCMOS25 [get_ports HDMI_R_D2]", "set_property PACKAGE_PIN D23 [get_ports HDMI_R_D3]", "set_property IOSTANDARD LVCMOS25 [get_ports HDMI_R_D3]", "set_property PACKAGE_PIN F25 [get_ports HDMI_R_D4]", "set_property IOSTANDARD LVCMOS25 [get_ports HDMI_R_D4]", "set_property PACKAGE_PIN E25 [get_ports HDMI_R_D5]", "set_property IOSTANDARD LVCMOS25 [get_ports HDMI_R_D5]", "set_property PACKAGE_PIN E24 [get_ports HDMI_R_D6]", "set_property IOSTANDARD LVCMOS25 [get_ports HDMI_R_D6]", "set_property PACKAGE_PIN D24 [get_ports HDMI_R_D7]", "set_property IOSTANDARD LVCMOS25 [get_ports HDMI_R_D7]", "set_property PACKAGE_PIN F26 [get_ports HDMI_R_D8]", "set_property IOSTANDARD LVCMOS25 [get_ports HDMI_R_D8]", "set_property PACKAGE_PIN E26 [get_ports HDMI_R_D9]", "set_property IOSTANDARD LVCMOS25 [get_ports HDMI_R_D9]", "set_property PACKAGE_PIN G23 [get_ports HDMI_R_D10]", "set_property IOSTANDARD LVCMOS25 [get_ports HDMI_R_D10]", "set_property PACKAGE_PIN G24 [get_ports HDMI_R_D11]", "set_property IOSTANDARD LVCMOS25 [get_ports HDMI_R_D11]", "set_property PACKAGE_PIN B27 [get_ports FMC_HPC_LA16_P]", "set_property IOSTANDARD LVCMOS25 [get_ports FMC_HPC_LA16_P]", "set_property PACKAGE_PIN A27 [get_ports FMC_HPC_LA16_N]", "set_property IOSTANDARD LVCMOS25 [get_ports FMC_HPC_LA16_N]", "set_property PACKAGE_PIN C24 [get_ports FMC_HPC_LA15_P]", "set_property IOSTANDARD LVCMOS25 [get_ports FMC_HPC_LA15_P]", "set_property PACKAGE_PIN B24 [get_ports FMC_HPC_LA15_N]", "set_property IOSTANDARD LVCMOS25 [get_ports FMC_HPC_LA15_N]", "set_property PACKAGE_PIN B28 [get_ports FMC_HPC_LA14_P]", "set_property IOSTANDARD LVCMOS25 [get_ports FMC_HPC_LA14_P]", "set_property PACKAGE_PIN A28 [get_ports FMC_HPC_LA14_N]", "set_property IOSTANDARD LVCMOS25 [get_ports FMC_HPC_LA14_N]", "set_property PACKAGE_PIN A25 [get_ports FMC_HPC_LA13_P]", "set_property IOSTANDARD LVCMOS25 [get_ports FMC_HPC_LA13_P]", "set_property PACKAGE_PIN A26 [get_ports FMC_HPC_LA13_N]", "set_property IOSTANDARD LVCMOS25 [get_ports FMC_HPC_LA13_N]", "set_property PACKAGE_PIN D26 [get_ports FMC_HPC_LA01_CC_P]", "set_property IOSTANDARD LVCMOS25 [get_ports FMC_HPC_LA01_CC_P]", "set_property PACKAGE_PIN C26 [get_ports FMC_HPC_LA01_CC_N]", "set_property IOSTANDARD LVCMOS25 [get_ports FMC_HPC_LA01_CC_N]", "set_property PACKAGE_PIN C25 [get_ports FMC_HPC_LA00_CC_P]", "set_property IOSTANDARD LVCMOS25 [get_ports FMC_HPC_LA00_CC_P]", "set_property PACKAGE_PIN B25 [get_ports FMC_HPC_LA00_CC_N]", "set_property IOSTANDARD LVCMOS25 [get_ports FMC_HPC_LA00_CC_N]", "set_property PACKAGE_PIN D27 [get_ports FMC_HPC_CLK0_M2C_P]", "set_property IOSTANDARD LVCMOS25 [get_ports FMC_HPC_CLK0_M2C_P]", "set_property PACKAGE_PIN C27 [get_ports FMC_HPC_CLK0_M2C_N]", "set_property IOSTANDARD LVCMOS25 [get_ports FMC_HPC_CLK0_M2C_N]", "set_property PACKAGE_PIN E28 [get_ports FMC_HPC_LA07_P]", "set_property IOSTANDARD LVCMOS25 [get_ports FMC_HPC_LA07_P]", "set_property PACKAGE_PIN D28 [get_ports FMC_HPC_LA07_N]", "set_property IOSTANDARD LVCMOS25 [get_ports FMC_HPC_LA07_N]", "set_property PACKAGE_PIN C29 [get_ports FMC_HPC_LA12_P]", "set_property IOSTANDARD LVCMOS25 [get_ports FMC_HPC_LA12_P]", "set_property PACKAGE_PIN B29 [get_ports FMC_HPC_LA12_N]", "set_property IOSTANDARD LVCMOS25 [get_ports FMC_HPC_LA12_N]", "set_property PACKAGE_PIN D29 [get_ports FMC_HPC_LA10_P]", "set_property IOSTANDARD LVCMOS25 [get_ports FMC_HPC_LA10_P]", "set_property PACKAGE_PIN C30 [get_ports FMC_HPC_LA10_N]", "set_property IOSTANDARD LVCMOS25 [get_ports FMC_HPC_LA10_N]", "set_property PACKAGE_PIN B30 [get_ports FMC_HPC_LA09_P]", "set_property IOSTANDARD LVCMOS25 [get_ports FMC_HPC_LA09_P]", "set_property PACKAGE_PIN A30 [get_ports FMC_HPC_LA09_N]", "set_property IOSTANDARD LVCMOS25 [get_ports FMC_HPC_LA09_N]", "set_property PACKAGE_PIN E29 [get_ports FMC_HPC_LA08_P]", "set_property IOSTANDARD LVCMOS25 [get_ports FMC_HPC_LA08_P]", "set_property PACKAGE_PIN E30 [get_ports FMC_HPC_LA08_N]", "set_property IOSTANDARD LVCMOS25 [get_ports FMC_HPC_LA08_N]", "set_property PACKAGE_PIN H24 [get_ports FMC_HPC_LA02_P]", "set_property IOSTANDARD LVCMOS25 [get_ports FMC_HPC_LA02_P]", "set_property PACKAGE_PIN H25 [get_ports FMC_HPC_LA02_N]", "set_property IOSTANDARD LVCMOS25 [get_ports FMC_HPC_LA02_N]", "set_property PACKAGE_PIN G28 [get_ports FMC_HPC_LA04_P]", "set_property IOSTANDARD LVCMOS25 [get_ports FMC_HPC_LA04_P]", "set_property PACKAGE_PIN F28 [get_ports FMC_HPC_LA04_N]", "set_property IOSTANDARD LVCMOS25 [get_ports FMC_HPC_LA04_N]", "set_property PACKAGE_PIN G27 [get_ports FMC_HPC_LA11_P]", "set_property IOSTANDARD LVCMOS25 [get_ports FMC_HPC_LA11_P]", "set_property PACKAGE_PIN F27 [get_ports FMC_HPC_LA11_N]", "set_property IOSTANDARD LVCMOS25 [get_ports FMC_HPC_LA11_N]", "set_property PACKAGE_PIN G29 [get_ports FMC_HPC_LA05_P]", "set_property IOSTANDARD LVCMOS25 [get_ports FMC_HPC_LA05_P]", "set_property PACKAGE_PIN F30 [get_ports FMC_HPC_LA05_N]", "set_property IOSTANDARD LVCMOS25 [get_ports FMC_HPC_LA05_N]", "set_property PACKAGE_PIN H26 [get_ports FMC_HPC_LA03_P]", "set_property IOSTANDARD LVCMOS25 [get_ports FMC_HPC_LA03_P]", "set_property PACKAGE_PIN H27 [get_ports FMC_HPC_LA03_N]", "set_property IOSTANDARD LVCMOS25 [get_ports FMC_HPC_LA03_N]", "set_property PACKAGE_PIN H30 [get_ports FMC_HPC_LA06_P]", "set_property IOSTANDARD LVCMOS25 [get_ports FMC_HPC_LA06_P]", "set_property PACKAGE_PIN G30 [get_ports FMC_HPC_LA06_N]", "set_property IOSTANDARD LVCMOS25 [get_ports FMC_HPC_LA06_N]", "set_property PACKAGE_PIN G25 [get_ports PCIE_PERST_LS]", "set_property IOSTANDARD LVCMOS25 [get_ports PCIE_PERST_LS]", "set_property PACKAGE_PIN G19 [get_ports GPIO_LED_5_LS]", "set_property IOSTANDARD LVCMOS25 [get_ports GPIO_LED_5_LS]", "set_property PACKAGE_PIN K18 [get_ports HDMI_R_CLK]", "set_property IOSTANDARD LVCMOS25 [get_ports HDMI_R_CLK]", "set_property PACKAGE_PIN J18 [get_ports HDMI_R_HSYNC]", "set_property IOSTANDARD LVCMOS25 [get_ports HDMI_R_HSYNC]", "set_property PACKAGE_PIN H20 [get_ports HDMI_R_VSYNC]", "set_property IOSTANDARD LVCMOS25 [get_ports HDMI_R_VSYNC]", "set_property PACKAGE_PIN G20 [get_ports HDMI_SPDIF_OUT_LS]", "set_property IOSTANDARD LVCMOS25 [get_ports HDMI_SPDIF_OUT_LS]", "set_property PACKAGE_PIN J17 [get_ports HDMI_R_SPDIF]", "set_property IOSTANDARD LVCMOS25 [get_ports HDMI_R_SPDIF]", "set_property PACKAGE_PIN H17 [get_ports HDMI_R_DE]", "set_property IOSTANDARD LVCMOS25 [get_ports HDMI_R_DE]", "set_property PACKAGE_PIN J19 [get_ports HDMI_R_D12]", "set_property IOSTANDARD LVCMOS25 [get_ports HDMI_R_D12]", "set_property PACKAGE_PIN H19 [get_ports HDMI_R_D13]", "set_property IOSTANDARD LVCMOS25 [get_ports HDMI_R_D13]", "set_property PACKAGE_PIN L17 [get_ports HDMI_R_D14]", "set_property IOSTANDARD LVCMOS25 [get_ports HDMI_R_D14]", "set_property PACKAGE_PIN L18 [get_ports HDMI_R_D15]", "set_property IOSTANDARD LVCMOS25 [get_ports HDMI_R_D15]", "set_property PACKAGE_PIN K19 [get_ports HDMI_R_D16]", "set_property IOSTANDARD LVCMOS25 [get_ports HDMI_R_D16]", "set_property PACKAGE_PIN K20 [get_ports HDMI_R_D17]", "set_property IOSTANDARD LVCMOS25 [get_ports HDMI_R_D17]", "set_property PACKAGE_PIN H21 [get_ports FMC_HPC_LA33_P]", "set_property IOSTANDARD LVCMOS25 [get_ports FMC_HPC_LA33_P]", "set_property PACKAGE_PIN H22 [get_ports FMC_HPC_LA33_N]", "set_property IOSTANDARD LVCMOS25 [get_ports FMC_HPC_LA33_N]", "set_property PACKAGE_PIN D21 [get_ports FMC_HPC_LA32_P]", "set_property IOSTANDARD LVCMOS25 [get_ports FMC_HPC_LA32_P]", "set_property PACKAGE_PIN C21 [get_ports FMC_HPC_LA32_N]", "set_property IOSTANDARD LVCMOS25 [get_ports FMC_HPC_LA32_N]", "set_property PACKAGE_PIN G22 [get_ports FMC_HPC_LA31_P]", "set_property IOSTANDARD LVCMOS25 [get_ports FMC_HPC_LA31_P]", "set_property PACKAGE_PIN F22 [get_ports FMC_HPC_LA31_N]", "set_property IOSTANDARD LVCMOS25 [get_ports FMC_HPC_LA31_N]", "set_property PACKAGE_PIN D22 [get_ports FMC_HPC_LA30_P]", "set_property IOSTANDARD LVCMOS25 [get_ports FMC_HPC_LA30_P]", "set_property PACKAGE_PIN C22 [get_ports FMC_HPC_LA30_N]", "set_property IOSTANDARD LVCMOS25 [get_ports FMC_HPC_LA30_N]", "set_property PACKAGE_PIN F21 [get_ports FMC_HPC_LA18_CC_P]", "set_property IOSTANDARD LVCMOS25 [get_ports FMC_HPC_LA18_CC_P]", "set_property PACKAGE_PIN E21 [get_ports FMC_HPC_LA18_CC_N]", "set_property IOSTANDARD LVCMOS25 [get_ports FMC_HPC_LA18_CC_N]", "set_property PACKAGE_PIN F20 [get_ports FMC_HPC_LA17_CC_P]", "set_property IOSTANDARD LVCMOS25 [get_ports FMC_HPC_LA17_CC_P]", "set_property PACKAGE_PIN E20 [get_ports FMC_HPC_LA17_CC_N]", "set_property IOSTANDARD LVCMOS25 [get_ports FMC_HPC_LA17_CC_N]", "set_property PACKAGE_PIN D17 [get_ports FMC_HPC_CLK1_M2C_P]", "set_property IOSTANDARD LVCMOS25 [get_ports FMC_HPC_CLK1_M2C_P]", "set_property PACKAGE_PIN D18 [get_ports FMC_HPC_CLK1_M2C_N]", "set_property IOSTANDARD LVCMOS25 [get_ports FMC_HPC_CLK1_M2C_N]", "set_property PACKAGE_PIN E19 [get_ports FMC_HPC_LA20_P]", "set_property IOSTANDARD LVCMOS25 [get_ports FMC_HPC_LA20_P]", "set_property PACKAGE_PIN D19 [get_ports FMC_HPC_LA20_N]", "set_property IOSTANDARD LVCMOS25 [get_ports FMC_HPC_LA20_N]", "set_property PACKAGE_PIN D16 [get_ports FMC_HPC_LA28_P]", "set_property IOSTANDARD LVCMOS25 [get_ports FMC_HPC_LA28_P]", "set_property PACKAGE_PIN C16 [get_ports FMC_HPC_LA28_N]", "set_property IOSTANDARD LVCMOS25 [get_ports FMC_HPC_LA28_N]", "set_property PACKAGE_PIN G18 [get_ports FMC_HPC_LA19_P]", "set_property IOSTANDARD LVCMOS25 [get_ports FMC_HPC_LA19_P]", "set_property PACKAGE_PIN F18 [get_ports FMC_HPC_LA19_N]", "set_property IOSTANDARD LVCMOS25 [get_ports FMC_HPC_LA19_N]", "set_property PACKAGE_PIN C17 [get_ports FMC_HPC_LA29_P]", "set_property IOSTANDARD LVCMOS25 [get_ports FMC_HPC_LA29_P]", "set_property PACKAGE_PIN B17 [get_ports FMC_HPC_LA29_N]", "set_property IOSTANDARD LVCMOS25 [get_ports FMC_HPC_LA29_N]", "set_property PACKAGE_PIN G17 [get_ports FMC_HPC_LA25_P]", "set_property IOSTANDARD LVCMOS25 [get_ports FMC_HPC_LA25_P]", "set_property PACKAGE_PIN F17 [get_ports FMC_HPC_LA25_N]", "set_property IOSTANDARD LVCMOS25 [get_ports FMC_HPC_LA25_N]", "set_property PACKAGE_PIN C20 [get_ports FMC_HPC_LA22_P]", "set_property IOSTANDARD LVCMOS25 [get_ports FMC_HPC_LA22_P]", "set_property PACKAGE_PIN B20 [get_ports FMC_HPC_LA22_N]", "set_property IOSTANDARD LVCMOS25 [get_ports FMC_HPC_LA22_N]", "set_property PACKAGE_PIN A16 [get_ports FMC_HPC_LA24_P]", "set_property IOSTANDARD LVCMOS25 [get_ports FMC_HPC_LA24_P]", "set_property PACKAGE_PIN A17 [get_ports FMC_HPC_LA24_N]", "set_property IOSTANDARD LVCMOS25 [get_ports FMC_HPC_LA24_N]", "set_property PACKAGE_PIN A20 [get_ports FMC_HPC_LA21_P]", "set_property IOSTANDARD LVCMOS25 [get_ports FMC_HPC_LA21_P]", "set_property PACKAGE_PIN A21 [get_ports FMC_HPC_LA21_N]", "set_property IOSTANDARD LVCMOS25 [get_ports FMC_HPC_LA21_N]", "set_property PACKAGE_PIN B18 [get_ports FMC_HPC_LA26_P]", "set_property IOSTANDARD LVCMOS25 [get_ports FMC_HPC_LA26_P]", "set_property PACKAGE_PIN A18 [get_ports FMC_HPC_LA26_N]", "set_property IOSTANDARD LVCMOS25 [get_ports FMC_HPC_LA26_N]", "set_property PACKAGE_PIN B22 [get_ports FMC_HPC_LA23_P]", "set_property IOSTANDARD LVCMOS25 [get_ports FMC_HPC_LA23_P]", "set_property PACKAGE_PIN A22 [get_ports FMC_HPC_LA23_N]", "set_property IOSTANDARD LVCMOS25 [get_ports FMC_HPC_LA23_N]", "set_property PACKAGE_PIN C19 [get_ports FMC_HPC_LA27_P]", "set_property IOSTANDARD LVCMOS25 [get_ports FMC_HPC_LA27_P]", "set_property PACKAGE_PIN B19 [get_ports FMC_HPC_LA27_N]", "set_property IOSTANDARD LVCMOS25 [get_ports FMC_HPC_LA27_N]", "set_property PACKAGE_PIN E18 [get_ports GPIO_LED_6_LS]", "set_property IOSTANDARD LVCMOS25 [get_ports GPIO_LED_6_LS]", "set_property PACKAGE_PIN G12 [get_ports GPIO_SW_C]", "set_property IOSTANDARD LVCMOS25 [get_ports GPIO_SW_C]", "set_property PACKAGE_PIN L16 [get_ports FMC_HPC_HA13_P]", "set_property IOSTANDARD LVCMOS25 [get_ports FMC_HPC_HA13_P]", "set_property PACKAGE_PIN K16 [get_ports FMC_HPC_HA13_N]", "set_property IOSTANDARD LVCMOS25 [get_ports FMC_HPC_HA13_N]", "set_property PACKAGE_PIN L15 [get_ports FMC_HPC_HA16_P]", "set_property IOSTANDARD LVCMOS25 [get_ports FMC_HPC_HA16_P]", "set_property PACKAGE_PIN K15 [get_ports FMC_HPC_HA16_N]", "set_property IOSTANDARD LVCMOS25 [get_ports FMC_HPC_HA16_N]", "set_property PACKAGE_PIN L12 [get_ports FMC_HPC_HA23_P]", "set_property IOSTANDARD LVCMOS25 [get_ports FMC_HPC_HA23_P]", "set_property PACKAGE_PIN L13 [get_ports FMC_HPC_HA23_N]", "set_property IOSTANDARD LVCMOS25 [get_ports FMC_HPC_HA23_N]", "set_property PACKAGE_PIN K13 [get_ports FMC_HPC_HA20_P]", "set_property IOSTANDARD LVCMOS25 [get_ports FMC_HPC_HA20_P]", "set_property PACKAGE_PIN J13 [get_ports FMC_HPC_HA20_N]", "set_property IOSTANDARD LVCMOS25 [get_ports FMC_HPC_HA20_N]", "set_property PACKAGE_PIN K14 [get_ports FMC_HPC_HA18_P]", "set_property IOSTANDARD LVCMOS25 [get_ports FMC_HPC_HA18_P]", "set_property PACKAGE_PIN J14 [get_ports FMC_HPC_HA18_N]", "set_property IOSTANDARD LVCMOS25 [get_ports FMC_HPC_HA18_N]", "set_property PACKAGE_PIN L11 [get_ports FMC_HPC_HA22_P]", "set_property IOSTANDARD LVCMOS25 [get_ports FMC_HPC_HA22_P]", "set_property PACKAGE_PIN K11 [get_ports FMC_HPC_HA22_N]", "set_property IOSTANDARD LVCMOS25 [get_ports FMC_HPC_HA22_N]", "set_property PACKAGE_PIN H15 [get_ports FMC_HPC_HA15_P]", "set_property IOSTANDARD LVCMOS25 [get_ports FMC_HPC_HA15_P]", "set_property PACKAGE_PIN G15 [get_ports FMC_HPC_HA15_N]", "set_property IOSTANDARD LVCMOS25 [get_ports FMC_HPC_HA15_N]", "set_property PACKAGE_PIN J11 [get_ports FMC_HPC_HA21_P]", "set_property IOSTANDARD LVCMOS25 [get_ports FMC_HPC_HA21_P]", "set_property PACKAGE_PIN J12 [get_ports FMC_HPC_HA21_N]", "set_property IOSTANDARD LVCMOS25 [get_ports FMC_HPC_HA21_N]", "set_property PACKAGE_PIN J16 [get_ports FMC_HPC_HA14_P]", "set_property IOSTANDARD LVCMOS25 [get_ports FMC_HPC_HA14_P]", "set_property PACKAGE_PIN H16 [get_ports FMC_HPC_HA14_N]", "set_property IOSTANDARD LVCMOS25 [get_ports FMC_HPC_HA14_N]", "set_property PACKAGE_PIN H11 [get_ports FMC_HPC_HA19_P]", "set_property IOSTANDARD LVCMOS25 [get_ports FMC_HPC_HA19_P]", "set_property PACKAGE_PIN H12 [get_ports FMC_HPC_HA19_N]", "set_property IOSTANDARD LVCMOS25 [get_ports FMC_HPC_HA19_N]", "set_property PACKAGE_PIN H14 [get_ports FMC_HPC_HA01_CC_P]", "set_property IOSTANDARD LVCMOS25 [get_ports FMC_HPC_HA01_CC_P]", "set_property PACKAGE_PIN G14 [get_ports FMC_HPC_HA01_CC_N]", "set_property IOSTANDARD LVCMOS25 [get_ports FMC_HPC_HA01_CC_N]", "set_property PACKAGE_PIN G13 [get_ports FMC_HPC_HA17_CC_P]", "set_property IOSTANDARD LVCMOS25 [get_ports FMC_HPC_HA17_CC_P]", "set_property PACKAGE_PIN F13 [get_ports FMC_HPC_HA17_CC_N]", "set_property IOSTANDARD LVCMOS25 [get_ports FMC_HPC_HA17_CC_N]", "set_property PACKAGE_PIN D12 [get_ports FMC_HPC_HA00_CC_P]", "set_property IOSTANDARD LVCMOS25 [get_ports FMC_HPC_HA00_CC_P]", "set_property PACKAGE_PIN D13 [get_ports FMC_HPC_HA00_CC_N]", "set_property IOSTANDARD LVCMOS25 [get_ports FMC_HPC_HA00_CC_N]", "set_property PACKAGE_PIN F12 [get_ports FMC_HPC_HA09_P]", "set_property IOSTANDARD LVCMOS25 [get_ports FMC_HPC_HA09_P]", "set_property PACKAGE_PIN E13 [get_ports FMC_HPC_HA09_N]", "set_property IOSTANDARD LVCMOS25 [get_ports FMC_HPC_HA09_N]", "set_property PACKAGE_PIN C12 [get_ports FMC_HPC_HA03_P]", "set_property IOSTANDARD LVCMOS25 [get_ports FMC_HPC_HA03_P]", "set_property PACKAGE_PIN B12 [get_ports FMC_HPC_HA03_N]", "set_property IOSTANDARD LVCMOS25 [get_ports FMC_HPC_HA03_N]", "set_property PACKAGE_PIN F11 [get_ports FMC_HPC_HA04_P]", "set_property IOSTANDARD LVCMOS25 [get_ports FMC_HPC_HA04_P]", "set_property PACKAGE_PIN E11 [get_ports FMC_HPC_HA04_N]", "set_property IOSTANDARD LVCMOS25 [get_ports FMC_HPC_HA04_N]", "set_property PACKAGE_PIN A11 [get_ports FMC_HPC_HA10_P]", "set_property IOSTANDARD LVCMOS25 [get_ports FMC_HPC_HA10_P]", "set_property PACKAGE_PIN A12 [get_ports FMC_HPC_HA10_N]", "set_property IOSTANDARD LVCMOS25 [get_ports FMC_HPC_HA10_N]", "set_property PACKAGE_PIN D11 [get_ports FMC_HPC_HA02_P]", "set_property IOSTANDARD LVCMOS25 [get_ports FMC_HPC_HA02_P]", "set_property PACKAGE_PIN C11 [get_ports FMC_HPC_HA02_N]", "set_property IOSTANDARD LVCMOS25 [get_ports FMC_HPC_HA02_N]", "set_property PACKAGE_PIN F15 [get_ports FMC_HPC_HA05_P]", "set_property IOSTANDARD LVCMOS25 [get_ports FMC_HPC_HA05_P]", "set_property PACKAGE_PIN E16 [get_ports FMC_HPC_HA05_N]", "set_property IOSTANDARD LVCMOS25 [get_ports FMC_HPC_HA05_N]", "set_property PACKAGE_PIN E14 [get_ports FMC_HPC_HA08_P]", "set_property IOSTANDARD LVCMOS25 [get_ports FMC_HPC_HA08_P]", "set_property PACKAGE_PIN E15 [get_ports FMC_HPC_HA08_N]", "set_property IOSTANDARD LVCMOS25 [get_ports FMC_HPC_HA08_N]", "set_property PACKAGE_PIN D14 [get_ports FMC_HPC_HA06_P]", "set_property IOSTANDARD LVCMOS25 [get_ports FMC_HPC_HA06_P]", "set_property PACKAGE_PIN C14 [get_ports FMC_HPC_HA06_N]", "set_property IOSTANDARD LVCMOS25 [get_ports FMC_HPC_HA06_N]", "set_property PACKAGE_PIN B13 [get_ports FMC_HPC_HA11_P]", "set_property IOSTANDARD LVCMOS25 [get_ports FMC_HPC_HA11_P]", "set_property PACKAGE_PIN A13 [get_ports FMC_HPC_HA11_N]", "set_property IOSTANDARD LVCMOS25 [get_ports FMC_HPC_HA11_N]", "set_property PACKAGE_PIN C15 [get_ports FMC_HPC_HA12_P]", "set_property IOSTANDARD LVCMOS25 [get_ports FMC_HPC_HA12_P]", "set_property PACKAGE_PIN B15 [get_ports FMC_HPC_HA12_N]", "set_property IOSTANDARD LVCMOS25 [get_ports FMC_HPC_HA12_N]", "set_property PACKAGE_PIN B14 [get_ports FMC_HPC_HA07_P]", "set_property IOSTANDARD LVCMOS25 [get_ports FMC_HPC_HA07_P]", "set_property PACKAGE_PIN A15 [get_ports FMC_HPC_HA07_N]", "set_property IOSTANDARD LVCMOS25 [get_ports FMC_HPC_HA07_N]", "set_property PACKAGE_PIN F16 [get_ports GPIO_LED_7_LS]", "set_property IOSTANDARD LVCMOS25 [get_ports GPIO_LED_7_LS]", "set_property PACKAGE_PIN Y14 [get_ports PMBUS_DATA_LS]", "set_property IOSTANDARD LVCMOS15 [get_ports PMBUS_DATA_LS]", "set_property PACKAGE_PIN AK16 [get_ports DDR3_D24]", "set_property IOSTANDARD SSTL15 [get_ports DDR3_D24]", "set_property PACKAGE_PIN AK15 [get_ports DDR3_D31]", "set_property IOSTANDARD SSTL15 [get_ports DDR3_D31]", "set_property PACKAGE_PIN AG15 [get_ports DDR3_D26]", "set_property IOSTANDARD SSTL15 [get_ports DDR3_D26]", "set_property PACKAGE_PIN AH15 [get_ports DDR3_D30]", "set_property IOSTANDARD SSTL15 [get_ports DDR3_D30]", "set_property PACKAGE_PIN AH16 [get_ports DDR3_DQS3_P]", "set_property IOSTANDARD SSTL15 [get_ports DDR3_DQS3_P]", "set_property PACKAGE_PIN AJ16 [get_ports DDR3_DQS3_N]", "set_property IOSTANDARD SSTL15 [get_ports DDR3_DQS3_N]", "set_property PACKAGE_PIN AF15 [get_ports DDR3_D27]", "set_property IOSTANDARD SSTL15 [get_ports DDR3_D27]", "set_property PACKAGE_PIN AG14 [get_ports DDR3_D29]", "set_property IOSTANDARD SSTL15 [get_ports DDR3_D29]", "set_property PACKAGE_PIN AH17 [get_ports DDR3_D28]", "set_property IOSTANDARD SSTL15 [get_ports DDR3_D28]", "set_property PACKAGE_PIN AJ17 [get_ports DDR3_D25]", "set_property IOSTANDARD SSTL15 [get_ports DDR3_D25]", "set_property PACKAGE_PIN AE16 [get_ports DDR3_DM3]", "set_property IOSTANDARD SSTL15 [get_ports DDR3_DM3]", "set_property PACKAGE_PIN AF16 [get_ports VTTVREF]", "set_property PACKAGE_PIN AJ19 [get_ports DDR3_D21]", "set_property IOSTANDARD SSTL15 [get_ports DDR3_D21]", "set_property PACKAGE_PIN AK19 [get_ports DDR3_D17]", "set_property IOSTANDARD SSTL15 [get_ports DDR3_D17]", "set_property PACKAGE_PIN AG19 [get_ports DDR3_D16]", "set_property IOSTANDARD SSTL15 [get_ports DDR3_D16]", "set_property PACKAGE_PIN AH19 [get_ports DDR3_D20]", "set_property IOSTANDARD SSTL15 [get_ports DDR3_D20]", "set_property PACKAGE_PIN AJ18 [get_ports DDR3_DQS2_P]", "set_property IOSTANDARD SSTL15 [get_ports DDR3_DQS2_P]", "set_property PACKAGE_PIN AK18 [get_ports DDR3_DQS2_N]", "set_property IOSTANDARD SSTL15 [get_ports DDR3_DQS2_N]", "set_property PACKAGE_PIN AD19 [get_ports DDR3_D23]", "set_property IOSTANDARD SSTL15 [get_ports DDR3_D23]", "set_property PACKAGE_PIN AE19 [get_ports DDR3_D22]", "set_property IOSTANDARD SSTL15 [get_ports DDR3_D22]", "set_property PACKAGE_PIN AF18 [get_ports DDR3_D19]", "set_property IOSTANDARD SSTL15 [get_ports DDR3_D19]", "set_property PACKAGE_PIN AG18 [get_ports DDR3_D18]", "set_property IOSTANDARD SSTL15 [get_ports DDR3_D18]", "set_property PACKAGE_PIN AF17 [get_ports DDR3_DM2]", "set_property IOSTANDARD SSTL15 [get_ports DDR3_DM2]", "set_property PACKAGE_PIN AG17 [get_ports PMBUS_CLK_LS]", "set_property IOSTANDARD LVCMOS15 [get_ports PMBUS_CLK_LS]", "set_property PACKAGE_PIN AD18 [get_ports DDR3_D15]", "set_property IOSTANDARD SSTL15 [get_ports DDR3_D15]", "set_property PACKAGE_PIN AE18 [get_ports DDR3_D14]", "set_property IOSTANDARD SSTL15 [get_ports DDR3_D14]", "set_property PACKAGE_PIN AD17 [get_ports DDR3_D11]", "set_property IOSTANDARD SSTL15 [get_ports DDR3_D11]", "set_property PACKAGE_PIN AD16 [get_ports DDR3_D9]", "set_property IOSTANDARD SSTL15 [get_ports DDR3_D9]", "set_property PACKAGE_PIN Y19 [get_ports DDR3_DQS1_P]", "set_property IOSTANDARD DIFF_SSTL15 [get_ports DDR3_DQS1_P]", "set_property PACKAGE_PIN Y18 [get_ports DDR3_DQS1_N]", "set_property IOSTANDARD DIFF_SSTL15 [get_ports DDR3_DQS1_N]", "set_property PACKAGE_PIN AA18 [get_ports DDR3_D12]", "set_property IOSTANDARD SSTL15 [get_ports DDR3_D12]", "set_property PACKAGE_PIN AB18 [get_ports DDR3_D13]", "set_property IOSTANDARD SSTL15 [get_ports DDR3_D13]", "set_property PACKAGE_PIN AB19 [get_ports DDR3_D8]", "set_property IOSTANDARD SSTL15 [get_ports DDR3_D8]", "set_property PACKAGE_PIN AC19 [get_ports DDR3_D10]", "set_property IOSTANDARD SSTL15 [get_ports DDR3_D10]", "set_property PACKAGE_PIN AB17 [get_ports DDR3_DM1]", "set_property IOSTANDARD SSTL15 [get_ports DDR3_DM1]", "set_property PACKAGE_PIN AC17 [get_ports 7N700]", "set_property PACKAGE_PIN AE15 [get_ports DDR3_D6]", "set_property IOSTANDARD SSTL15 [get_ports DDR3_D6]", "set_property PACKAGE_PIN AE14 [get_ports VTTVREF]", "set_property PACKAGE_PIN AA15 [get_ports DDR3_D0]", "set_property IOSTANDARD SSTL15 [get_ports DDR3_D0]", "set_property PACKAGE_PIN AB15 [get_ports DDR3_D5]", "set_property IOSTANDARD SSTL15 [get_ports DDR3_D5]", "set_property PACKAGE_PIN AC16 [get_ports DDR3_DQS0_P]", "set_property IOSTANDARD DIFF_SSTL15 [get_ports DDR3_DQS0_P]", "set_property PACKAGE_PIN AC15 [get_ports DDR3_DQS0_N]", "set_property IOSTANDARD DIFF_SSTL15 [get_ports DDR3_DQS0_N]", "set_property PACKAGE_PIN AC14 [get_ports DDR3_D2]", "set_property IOSTANDARD SSTL15 [get_ports DDR3_D2]", "set_property PACKAGE_PIN AD14 [get_ports DDR3_D3]", "set_property IOSTANDARD SSTL15 [get_ports DDR3_D3]", "set_property PACKAGE_PIN AA17 [get_ports DDR3_D4]", "set_property IOSTANDARD SSTL15 [get_ports DDR3_D4]", "set_property PACKAGE_PIN AA16 [get_ports DDR3_D1]", "set_property IOSTANDARD SSTL15 [get_ports DDR3_D1]", "set_property PACKAGE_PIN Y16 [get_ports DDR3_DM0]", "set_property IOSTANDARD SSTL15 [get_ports DDR3_DM0]", "set_property PACKAGE_PIN Y15 [get_ports DDR3_D7]", "set_property IOSTANDARD SSTL15 [get_ports DDR3_D7]", "set_property PACKAGE_PIN AB14 [get_ports PMBUS_ALERT_LS]", "set_property IOSTANDARD LVCMOS15 [get_ports PMBUS_ALERT_LS]", "set_property PACKAGE_PIN Y13 [get_ports VRN_33]", "set_property IOSTANDARD SSTL15 [get_ports VRN_33]", "set_property PACKAGE_PIN AA12 [get_ports GPIO_SW_N]", "set_property IOSTANDARD LVCMOS15 [get_ports GPIO_SW_N]", "set_property PACKAGE_PIN AB12 [get_ports GPIO_SW_S]", "set_property IOSTANDARD LVCMOS15 [get_ports GPIO_SW_S]", "set_property PACKAGE_PIN AA8 [get_ports GPIO_LED_1_LS]", "set_property IOSTANDARD LVCMOS15 [get_ports GPIO_LED_1_LS]", "set_property PACKAGE_PIN AB8 [get_ports GPIO_LED_0_LS]", "set_property IOSTANDARD LVCMOS15 [get_ports GPIO_LED_0_LS]", "set_property PACKAGE_PIN AB9 [get_ports GPIO_LED_3_LS]", "set_property IOSTANDARD LVCMOS15 [get_ports GPIO_LED_3_LS]", "set_property PACKAGE_PIN AC9 [get_ports GPIO_LED_2_LS]", "set_property IOSTANDARD LVCMOS15 [get_ports GPIO_LED_2_LS]", "set_property PACKAGE_PIN Y11 [get_ports LCD_RS_LS]", "set_property IOSTANDARD LVCMOS15 [get_ports LCD_RS_LS]", "set_property PACKAGE_PIN Y10 [get_ports LCD_DB7_LS]", "set_property IOSTANDARD LVCMOS15 [get_ports LCD_DB7_LS]", "set_property PACKAGE_PIN AA11 [get_ports LCD_DB6_LS]", "set_property IOSTANDARD LVCMOS15 [get_ports LCD_DB6_LS]", "set_property PACKAGE_PIN AA10 [get_ports LCD_DB5_LS]", "set_property IOSTANDARD LVCMOS15 [get_ports LCD_DB5_LS]", "set_property PACKAGE_PIN AA13 [get_ports LCD_DB4_LS]", "set_property IOSTANDARD LVCMOS15 [get_ports LCD_DB4_LS]", "set_property PACKAGE_PIN AB13 [get_ports LCD_RW_LS]", "set_property IOSTANDARD LVCMOS15 [get_ports LCD_RW_LS]", "set_property PACKAGE_PIN AB10 [get_ports LCD_E_LS]", "set_property IOSTANDARD LVCMOS15 [get_ports LCD_E_LS]", "set_property PACKAGE_PIN AC10 [get_ports DDR3_ODT1]", "set_property IOSTANDARD SSTL15 [get_ports DDR3_ODT1]", "set_property PACKAGE_PIN AD8 [get_ports DDR3_ODT0]", "set_property IOSTANDARD SSTL15 [get_ports DDR3_ODT0]", "set_property PACKAGE_PIN AE8 [get_ports DDR3_S1_B]", "set_property IOSTANDARD SSTL15 [get_ports DDR3_S1_B]", "set_property PACKAGE_PIN AC12 [get_ports DDR3_S0_B]", "set_property IOSTANDARD SSTL15 [get_ports DDR3_S0_B]", "set_property PACKAGE_PIN AC11 [get_ports DDR3_CAS_B]", "set_property IOSTANDARD SSTL15 [get_ports DDR3_CAS_B]", "set_property PACKAGE_PIN AD9 [get_ports DDR3_RAS_B]", "set_property IOSTANDARD SSTL15 [get_ports DDR3_RAS_B]", "set_property PACKAGE_PIN AE9 [get_ports DDR3_WE_B]", "set_property IOSTANDARD SSTL15 [get_ports DDR3_WE_B]", "set_property PACKAGE_PIN AE11 [get_ports DDR3_CLK1_P]", "set_property IOSTANDARD DIFF_SSTL15 [get_ports DDR3_CLK1_P]", "set_property PACKAGE_PIN AF11 [get_ports DDR3_CLK1_N]", "set_property IOSTANDARD DIFF_SSTL15 [get_ports DDR3_CLK1_N]", "set_property PACKAGE_PIN AD12 [get_ports SYSCLK_P]", "set_property IOSTANDARD LVDS [get_ports SYSCLK_P]", "set_property PACKAGE_PIN AD11 [get_ports SYSCLK_N]", "set_property IOSTANDARD LVDS [get_ports SYSCLK_N]", "set_property PACKAGE_PIN AG10 [get_ports DDR3_CLK0_P]", "set_property IOSTANDARD DIFF_SSTL15 [get_ports DDR3_CLK0_P]", "set_property PACKAGE_PIN AH10 [get_ports DDR3_CLK0_N]", "set_property IOSTANDARD DIFF_SSTL15 [get_ports DDR3_CLK0_N]", "set_property PACKAGE_PIN AE10 [get_ports DDR3_CKE1]", "set_property IOSTANDARD SSTL15 [get_ports DDR3_CKE1]", "set_property PACKAGE_PIN AF10 [get_ports DDR3_CKE0]", "set_property IOSTANDARD SSTL15 [get_ports DDR3_CKE0]", "set_property PACKAGE_PIN AJ9 [get_ports DDR3_TEMP_EVENT]", "set_property IOSTANDARD SSTL15 [get_ports DDR3_TEMP_EVENT]", "set_property PACKAGE_PIN AK9 [get_ports DDR3_BA2]", "set_property IOSTANDARD SSTL15 [get_ports DDR3_BA2]", "set_property PACKAGE_PIN AG9 [get_ports DDR3_BA1]", "set_property IOSTANDARD SSTL15 [get_ports DDR3_BA1]", "set_property PACKAGE_PIN AH9 [get_ports DDR3_BA0]", "set_property IOSTANDARD SSTL15 [get_ports DDR3_BA0]", "set_property PACKAGE_PIN AK11 [get_ports DDR3_A15]", "set_property IOSTANDARD SSTL15 [get_ports DDR3_A15]", "set_property PACKAGE_PIN AK10 [get_ports DDR3_A14]", "set_property IOSTANDARD SSTL15 [get_ports DDR3_A14]", "set_property PACKAGE_PIN AH11 [get_ports DDR3_A13]", "set_property IOSTANDARD SSTL15 [get_ports DDR3_A13]", "set_property PACKAGE_PIN AJ11 [get_ports DDR3_A12]", "set_property IOSTANDARD SSTL15 [get_ports DDR3_A12]", "set_property PACKAGE_PIN AE13 [get_ports DDR3_A11]", "set_property IOSTANDARD SSTL15 [get_ports DDR3_A11]", "set_property PACKAGE_PIN AF13 [get_ports DDR3_A10]", "set_property IOSTANDARD SSTL15 [get_ports DDR3_A10]", "set_property PACKAGE_PIN AK14 [get_ports DDR3_A9]", "set_property IOSTANDARD SSTL15 [get_ports DDR3_A9]", "set_property PACKAGE_PIN AK13 [get_ports DDR3_A8]", "set_property IOSTANDARD SSTL15 [get_ports DDR3_A8]", "set_property PACKAGE_PIN AH14 [get_ports DDR3_A7]", "set_property IOSTANDARD SSTL15 [get_ports DDR3_A7]", "set_property PACKAGE_PIN AJ14 [get_ports DDR3_A6]", "set_property IOSTANDARD SSTL15 [get_ports DDR3_A6]", "set_property PACKAGE_PIN AJ13 [get_ports DDR3_A5]", "set_property IOSTANDARD SSTL15 [get_ports DDR3_A5]", "set_property PACKAGE_PIN AJ12 [get_ports DDR3_A4]", "set_property IOSTANDARD SSTL15 [get_ports DDR3_A4]", "set_property PACKAGE_PIN AF12 [get_ports DDR3_A3]", "set_property IOSTANDARD SSTL15 [get_ports DDR3_A3]", "set_property PACKAGE_PIN AG12 [get_ports DDR3_A2]", "set_property IOSTANDARD SSTL15 [get_ports DDR3_A2]", "set_property PACKAGE_PIN AG13 [get_ports DDR3_A1]", "set_property IOSTANDARD SSTL15 [get_ports DDR3_A1]", "set_property PACKAGE_PIN AH12 [get_ports DDR3_A0]", "set_property IOSTANDARD SSTL15 [get_ports DDR3_A0]", "set_property PACKAGE_PIN AD13 [get_ports VRP_33]", "set_property PACKAGE_PIN AC6 [get_ports GPIO_SW_W]", "set_property IOSTANDARD LVCMOS15 [get_ports GPIO_SW_W]", "set_property PACKAGE_PIN AD4 [get_ports DDR3_D63]", "set_property IOSTANDARD SSTL15 [get_ports DDR3_D63]", "set_property PACKAGE_PIN AD3 [get_ports DDR3_D57]", "set_property IOSTANDARD SSTL15 [get_ports DDR3_D57]", "set_property PACKAGE_PIN AC2 [get_ports DDR3_D62]", "set_property IOSTANDARD SSTL15 [get_ports DDR3_D62]", "set_property PACKAGE_PIN AC1 [get_ports DDR3_D56]", "set_property IOSTANDARD SSTL15 [get_ports DDR3_D56]", "set_property PACKAGE_PIN AD2 [get_ports DDR3_DQS7_P]", "set_property IOSTANDARD DIFF_SSTL15 [get_ports DDR3_DQS7_P]", "set_property PACKAGE_PIN AD1 [get_ports DDR3_DQS7_N]", "set_property IOSTANDARD DIFF_SSTL15 [get_ports DDR3_DQS7_N]", "set_property PACKAGE_PIN AC5 [get_ports DDR3_D59]", "set_property IOSTANDARD SSTL15 [get_ports DDR3_D59]", "set_property PACKAGE_PIN AC4 [get_ports DDR3_D58]", "set_property IOSTANDARD SSTL15 [get_ports DDR3_D58]", "set_property PACKAGE_PIN AD6 [get_ports DDR3_D61]", "set_property IOSTANDARD SSTL15 [get_ports DDR3_D61]", "set_property PACKAGE_PIN AE6 [get_ports DDR3_D60]", "set_property IOSTANDARD SSTL15 [get_ports DDR3_D60]", "set_property PACKAGE_PIN AC7 [get_ports DDR3_DM7]", "set_property IOSTANDARD SSTL15 [get_ports DDR3_DM7]", "set_property PACKAGE_PIN AD7 [get_ports VTTVREF]", "set_property PACKAGE_PIN AF3 [get_ports DDR3_D52]", "set_property IOSTANDARD SSTL15 [get_ports DDR3_D52]", "set_property PACKAGE_PIN AF2 [get_ports DDR3_D49]", "set_property IOSTANDARD SSTL15 [get_ports DDR3_D49]", "set_property PACKAGE_PIN AE1 [get_ports DDR3_D54]", "set_property IOSTANDARD SSTL15 [get_ports DDR3_D54]", "set_property PACKAGE_PIN AF1 [get_ports DDR3_D48]", "set_property IOSTANDARD SSTL15 [get_ports DDR3_D48]", "set_property PACKAGE_PIN AG4 [get_ports DDR3_DQS6_P]", "set_property IOSTANDARD DIFF_SSTL15 [get_ports DDR3_DQS6_P]", "set_property PACKAGE_PIN AG3 [get_ports DDR3_DQS6_N]", "set_property IOSTANDARD DIFF_SSTL15 [get_ports DDR3_DQS6_N]", "set_property PACKAGE_PIN AE4 [get_ports DDR3_D50]", "set_property IOSTANDARD SSTL15 [get_ports DDR3_D50]", "set_property PACKAGE_PIN AE3 [get_ports DDR3_D51]", "set_property IOSTANDARD SSTL15 [get_ports DDR3_D51]", "set_property PACKAGE_PIN AE5 [get_ports DDR3_D55]", "set_property IOSTANDARD SSTL15 [get_ports DDR3_D55]", "set_property PACKAGE_PIN AF5 [get_ports DDR3_D53]", "set_property IOSTANDARD SSTL15 [get_ports DDR3_D53]", "set_property PACKAGE_PIN AF6 [get_ports DDR3_DM6]", "set_property IOSTANDARD SSTL15 [get_ports DDR3_DM6]", "set_property PACKAGE_PIN AG5 [get_ports GPIO_SW_E]", "set_property IOSTANDARD LVCMOS15 [get_ports GPIO_SW_E]", "set_property PACKAGE_PIN AH4 [get_ports DDR3_D44]", "set_property IOSTANDARD SSTL15 [get_ports DDR3_D44]", "set_property PACKAGE_PIN AJ4 [get_ports DDR3_D45]", "set_property IOSTANDARD SSTL15 [get_ports DDR3_D45]", "set_property PACKAGE_PIN AH6 [get_ports DDR3_D41]", "set_property IOSTANDARD SSTL15 [get_ports DDR3_D41]", "set_property PACKAGE_PIN AH5 [get_ports DDR3_D40]", "set_property IOSTANDARD SSTL15 [get_ports DDR3_D40]", "set_property PACKAGE_PIN AG2 [get_ports DDR3_DQS5_P]", "set_property IOSTANDARD DIFF_SSTL15 [get_ports DDR3_DQS5_P]", "set_property PACKAGE_PIN AH1 [get_ports DDR3_DQS5_N]", "set_property IOSTANDARD DIFF_SSTL15 [get_ports DDR3_DQS5_N]", "set_property PACKAGE_PIN AH2 [get_ports DDR3_D43]", "set_property IOSTANDARD SSTL15 [get_ports DDR3_D43]", "set_property PACKAGE_PIN AJ2 [get_ports DDR3_D42]", "set_property IOSTANDARD SSTL15 [get_ports DDR3_D42]", "set_property PACKAGE_PIN AJ1 [get_ports DDR3_D47]", "set_property IOSTANDARD SSTL15 [get_ports DDR3_D47]", "set_property PACKAGE_PIN AK1 [get_ports DDR3_D46]", "set_property IOSTANDARD SSTL15 [get_ports DDR3_D46]", "set_property PACKAGE_PIN AJ3 [get_ports DDR3_DM5]", "set_property IOSTANDARD SSTL15 [get_ports DDR3_DM5]", "set_property PACKAGE_PIN AK3 [get_ports DDR3_RESET_B]", "set_property IOSTANDARD LVCMOS15 [get_ports DDR3_RESET_B]", "set_property PACKAGE_PIN AF8 [get_ports DDR3_D36]", "set_property IOSTANDARD SSTL15 [get_ports DDR3_D36]", "set_property PACKAGE_PIN AG8 [get_ports VTTVREF]", "set_property PACKAGE_PIN AF7 [get_ports DDR3_D35]", "set_property IOSTANDARD SSTL15 [get_ports DDR3_D35]", "set_property PACKAGE_PIN AG7 [get_ports DDR3_D34]", "set_property IOSTANDARD SSTL15 [get_ports DDR3_D34]", "set_property PACKAGE_PIN AH7 [get_ports DDR3_DQS4_P]", "set_property IOSTANDARD DIFF_SSTL15 [get_ports DDR3_DQS4_P]", "set_property PACKAGE_PIN AJ7 [get_ports DDR3_DQS4_N]", "set_property IOSTANDARD DIFF_SSTL15 [get_ports DDR3_DQS4_N]", "set_property PACKAGE_PIN AJ6 [get_ports DDR3_D39]", "set_property IOSTANDARD SSTL15 [get_ports DDR3_D39]", "set_property PACKAGE_PIN AK6 [get_ports DDR3_D33]", "set_property IOSTANDARD SSTL15 [get_ports DDR3_D33]", "set_property PACKAGE_PIN AJ8 [get_ports DDR3_D38]", "set_property IOSTANDARD SSTL15 [get_ports DDR3_D38]", "set_property PACKAGE_PIN AK8 [get_ports DDR3_D32]", "set_property IOSTANDARD SSTL15 [get_ports DDR3_D32]", "set_property PACKAGE_PIN AK5 [get_ports DDR3_DM4]", "set_property IOSTANDARD SSTL15 [get_ports DDR3_DM4]", "set_property PACKAGE_PIN AK4 [get_ports DDR3_D37]", "set_property IOSTANDARD SSTL15 [get_ports DDR3_D37]", "set_property PACKAGE_PIN AB7 [get_ports CPU_RESET]", "set_property IOSTANDARD LVCMOS15 [get_ports CPU_RESET]", "set_property PACKAGE_PIN T2 [get_ports PCIE_TX4_P]", "set_property PACKAGE_PIN V6 [get_ports PCIE_RX4_P]", "set_property PACKAGE_PIN T1 [get_ports PCIE_TX4_N]", "set_property PACKAGE_PIN V5 [get_ports PCIE_RX4_N]", "set_property PACKAGE_PIN U4 [get_ports PCIE_TX5_P]", "set_property PACKAGE_PIN W4 [get_ports PCIE_RX5_P]", "set_property PACKAGE_PIN U3 [get_ports PCIE_TX5_N]", "set_property PACKAGE_PIN R8 [get_ports 9N302]", "set_property PACKAGE_PIN W3 [get_ports PCIE_RX5_N]", "set_property PACKAGE_PIN R7 [get_ports 9N301]", "set_property PACKAGE_PIN W8 [get_ports 9N173]", "set_property PACKAGE_PIN U7 [get_ports PCIE_CLK_QO_N]", "set_property PACKAGE_PIN U8 [get_ports PCIE_CLK_QO_P]", "set_property PACKAGE_PIN V2 [get_ports PCIE_TX6_P]", "set_property PACKAGE_PIN Y6 [get_ports PCIE_RX6_P]", "set_property PACKAGE_PIN V1 [get_ports PCIE_TX6_N]", "set_property PACKAGE_PIN Y5 [get_ports PCIE_RX6_N]", "set_property PACKAGE_PIN Y2 [get_ports PCIE_TX7_P]", "set_property PACKAGE_PIN AA4 [get_ports PCIE_RX7_P]", "set_property PACKAGE_PIN Y1 [get_ports PCIE_TX7_N]", "set_property PACKAGE_PIN AA3 [get_ports PCIE_RX7_N]", "set_property PACKAGE_PIN L4 [get_ports PCIE_TX0_P]", "set_property PACKAGE_PIN M6 [get_ports PCIE_RX0_P]", "set_property PACKAGE_PIN L3 [get_ports PCIE_TX0_N]", "set_property PACKAGE_PIN M5 [get_ports PCIE_RX0_N]", "set_property PACKAGE_PIN M2 [get_ports PCIE_TX1_P]", "set_property PACKAGE_PIN P6 [get_ports PCIE_RX1_P]", "set_property PACKAGE_PIN M1 [get_ports PCIE_TX1_N]", "set_property PACKAGE_PIN L8 [get_ports SI5326_OUT_C_P]", "set_property PACKAGE_PIN P5 [get_ports PCIE_RX1_N]", "set_property PACKAGE_PIN L7 [get_ports SI5326_OUT_C_N]", "set_property PACKAGE_PIN N7 [get_ports FMC_LPC_GBTCLK0_M2C_C_N]", "set_property PACKAGE_PIN N8 [get_ports FMC_LPC_GBTCLK0_M2C_C_P]", "set_property PACKAGE_PIN N4 [get_ports PCIE_TX2_P]", "set_property PACKAGE_PIN R4 [get_ports PCIE_RX2_P]", "set_property PACKAGE_PIN N3 [get_ports PCIE_TX2_N]", "set_property PACKAGE_PIN R3 [get_ports PCIE_RX2_N]", "set_property PACKAGE_PIN P2 [get_ports PCIE_TX3_P]", "set_property PACKAGE_PIN T6 [get_ports PCIE_RX3_P]", "set_property PACKAGE_PIN P1 [get_ports PCIE_TX3_N]", "set_property PACKAGE_PIN T5 [get_ports PCIE_RX3_N]", "set_property PACKAGE_PIN F2 [get_ports FMC_LPC_DP0_C2M_P]", "set_property PACKAGE_PIN F6 [get_ports FMC_LPC_DP0_M2C_P]", "set_property PACKAGE_PIN F1 [get_ports FMC_LPC_DP0_C2M_N]", "set_property PACKAGE_PIN F5 [get_ports FMC_LPC_DP0_M2C_N]", "set_property PACKAGE_PIN H2 [get_ports SFP_TX_P]", "set_property PACKAGE_PIN G4 [get_ports SFP_RX_N]", "set_property PACKAGE_PIN H1 [get_ports SFP_TX_N]", "set_property PACKAGE_PIN G8 [get_ports SGMIICLK_Q0_P]", "set_property PACKAGE_PIN G3 [get_ports SFP_RX_P]", "set_property PACKAGE_PIN G7 [get_ports SGMIICLK_Q0_N]", "set_property PACKAGE_PIN J7 [get_ports SMA_MGT_REFCLK_N]", "set_property PACKAGE_PIN J8 [get_ports SMA_MGT_REFCLK_P]", "set_property PACKAGE_PIN J4 [get_ports SGMII_TX_P]", "set_property PACKAGE_PIN H6 [get_ports SGMII_RX_P]", "set_property PACKAGE_PIN J3 [get_ports SGMII_TX_N]", "set_property PACKAGE_PIN H5 [get_ports SGMII_RX_N]", "set_property PACKAGE_PIN K2 [get_ports SMA_MGT_TX_P]", "set_property PACKAGE_PIN K6 [get_ports SMA_MGT_RX_P]", "set_property PACKAGE_PIN K1 [get_ports SMA_MGT_TX_N]", "set_property PACKAGE_PIN K5 [get_ports SMA_MGT_RX_N]", "set_property PACKAGE_PIN A4 [get_ports FMC_HPC_DP3_C2M_P]", "set_property PACKAGE_PIN A8 [get_ports FMC_HPC_DP3_M2C_P]", "set_property PACKAGE_PIN A3 [get_ports FMC_HPC_DP3_C2M_N]", "set_property PACKAGE_PIN A7 [get_ports FMC_HPC_DP3_M2C_N]", "set_property PACKAGE_PIN B2 [get_ports FMC_HPC_DP2_C2M_P]", "set_property PACKAGE_PIN B6 [get_ports FMC_HPC_DP2_M2C_P]", "set_property PACKAGE_PIN B1 [get_ports FMC_HPC_DP2_C2M_N]", "set_property PACKAGE_PIN C8 [get_ports FMC_HPC_GBTCLK0_M2C_C_P]", "set_property PACKAGE_PIN B5 [get_ports FMC_HPC_DP2_M2C_N]", "set_property PACKAGE_PIN C7 [get_ports FMC_HPC_GBTCLK0_M2C_C_N]", "set_property PACKAGE_PIN E7 [get_ports FMC_HPC_GBTCLK1_M2C_C_N]", "set_property PACKAGE_PIN E8 [get_ports FMC_HPC_GBTCLK1_M2C_C_P]", "set_property PACKAGE_PIN C4 [get_ports FMC_HPC_DP1_C2M_P]", "set_property PACKAGE_PIN D6 [get_ports FMC_HPC_DP1_M2C_P]", "set_property PACKAGE_PIN C3 [get_ports FMC_HPC_DP1_C2M_N]", "set_property PACKAGE_PIN D5 [get_ports FMC_HPC_DP1_M2C_N]", "set_property PACKAGE_PIN D2 [get_ports FMC_HPC_DP0_C2M_P]", "set_property PACKAGE_PIN E4 [get_ports FMC_HPC_DP0_M2C_P]", "set_property PACKAGE_PIN D1 [get_ports FMC_HPC_DP0_C2M_N]", "set_property PACKAGE_PIN E3 [get_ports FMC_HPC_DP0_M2C_N]"]
  in  "fmc":path=path "G:/tdc/2017/muon子板映射.csv"
  out "Array":string[][](array[string])=[["VO0", "HPC_LA02_N", "H25"], ["VO1", "HPC_HA06_N", "C14"], ["VO2", "HPC_HA10_N", "A12"], ["VO3", "HPC_HA15_N", "G15"], ["VO4", "HPC_LA20_N", "D19"], ["VO7", "HPC_LA24_N", "A17"], ["VO11", "HPC_HA08_N", "E15"], ["VO12", "HPC_HA12_N", "B15"], ["VO13", "HPC_HA20_N", "J13"], ["VO14", "HPC_LA19_N", "F18"], ["VO15", "HPC_LA23_N", "A22"], ["VO20", "HPC_HA09_N", "E13"], ["VO21", "HPC_HA13_N", "K16"], ["VO22", "HPC_HA16_N", "K15"], ["VO23", "HPC_LA15_N", "B24"], ["VO24", "HPC_HA23_N", "L13"], ["VO25", "HPC_LA21_N", "A21"], ["VO30", "HPC_HA07_N", "A15"], ["VO31", "HPC_LA05_N", "F30"], ["VO32", "HPC_LA10_N", "C30"], ["VO34", "HPC_HA22_N", "K11"], ["VO38", "HPC_LA31_N", "F22"], ["VO40", "HPC_LA03_N", "H27"], ["VO41", "HPC_LA08_N", "E30"], ["VO42", "HPC_HA14_N", "H16"], ["VO43", "HPC_HA18_N", "J14"], ["VO46", "HPC_LA25_N", "F17"], ["VO47", "HPC_LA28_N", "C16"], ["VO49", "HPC_LA32_N", "C21"], ["VO50", "HPC_LA04_N", "F28"], ["VO51", "HPC_HA11_N", "A13"], ["VO52", "HPC_LA09_N", "A30"], ["VO53", "HPC_HA19_N", "H12"], ["VO55", "HPC_LA27_N", "B19"], ["VO56", "HPC_LA26_N", "A18"], ["VO57", "HPC_LA29_N", "B17"], ["VO58", "HPC_LA30_N", "C22"], ["VO60", "HPC_LA06_N", "G30"], ["VO61", "HPC_LA07_N", "D28"], ["VO62", "HPC_LA12_N", "B29"], ["VO63", "HPC_HA21_N", "J12"]]
  in  "kc705_xdc":path=path "G:/fpga_tdc/PCB/KC705_Rev1_0_U1.ucf.xdc"
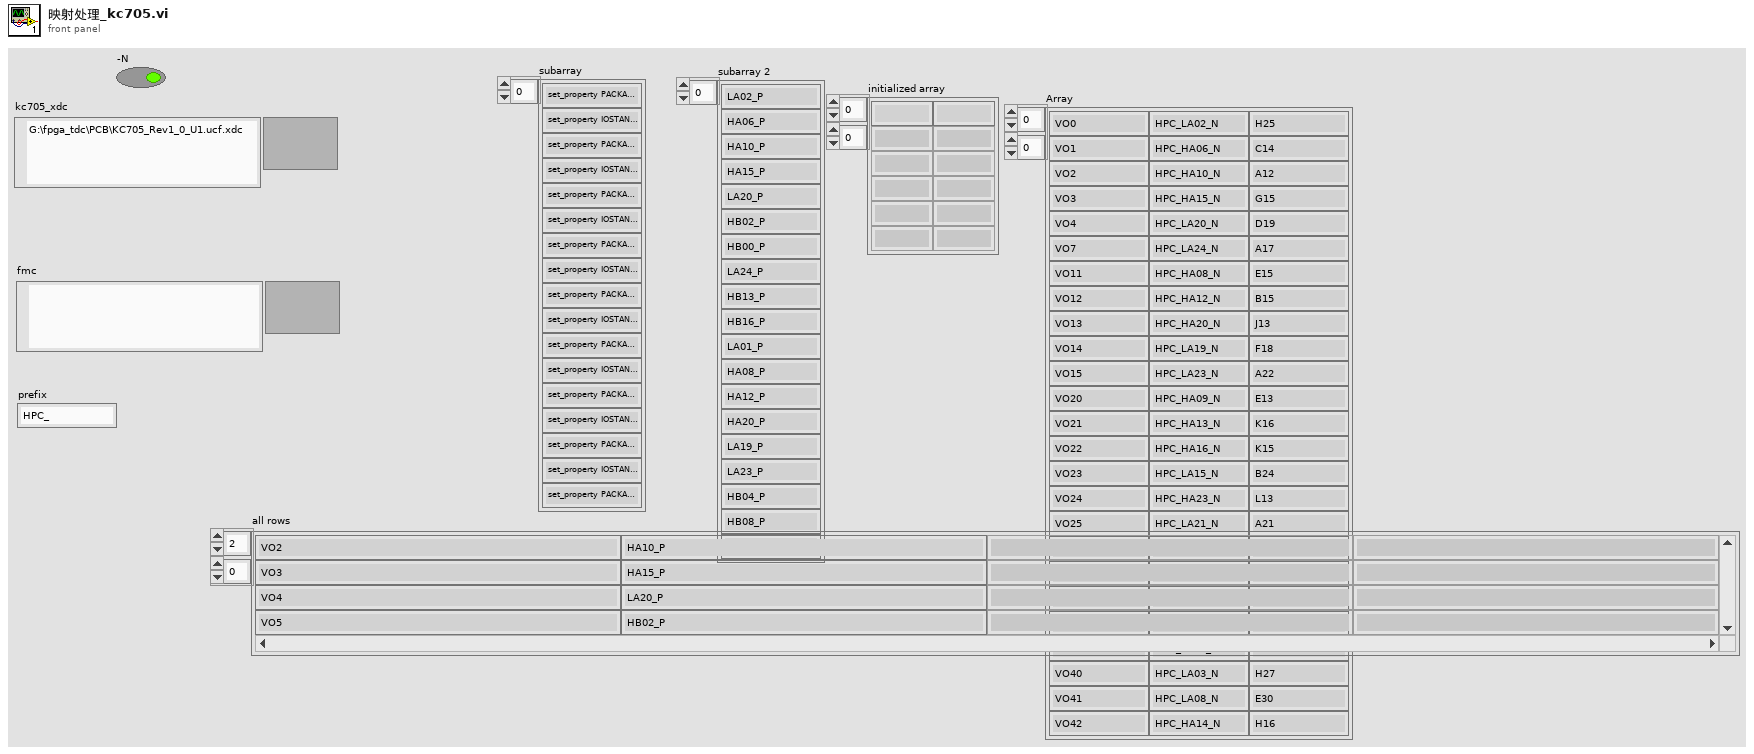
[diagram p1: front panel]
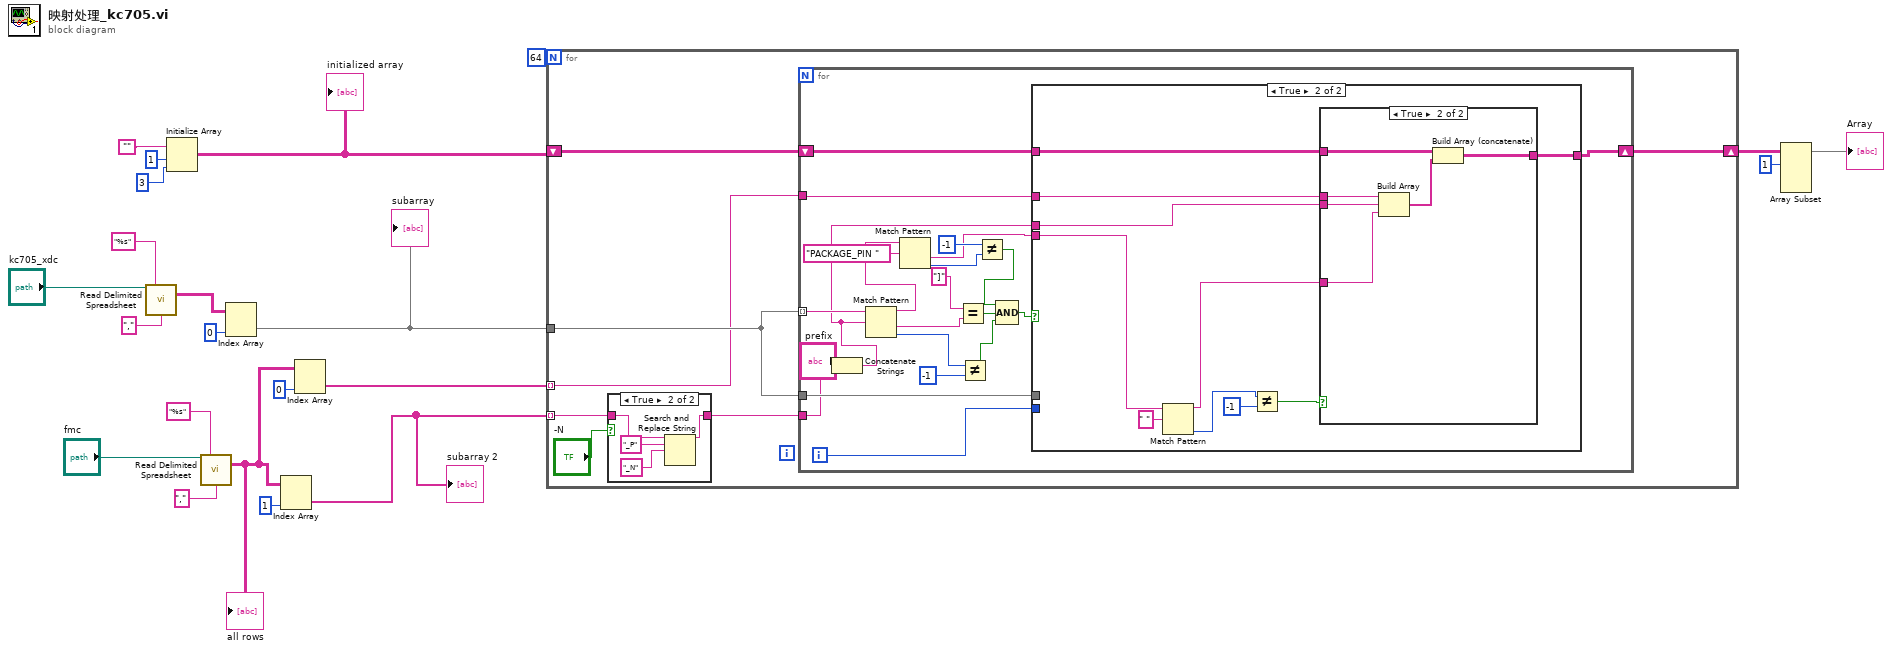
[diagram p0: block diagram]
diagram:
  n1 = call-poly <vilib>:"Read Delimited Spreadsheet.vi"("file path (dialog if empty)"="kc705_xdc", "format (%s)"="%s" ("format (%.3f)"), "delimiter (\\t)"="," ("delimiter (\\t)")) -> ("all rows"=w20:string[][])  [unwired: 7 in, 5 out]
  n2 = Initialize Array("", 1 ("dimension size"), 3 ("dimension size")) -> (w17:string[][])
  "initialized array" <- w17
  n3 = call-poly <vilib>:"Read Delimited Spreadsheet.vi"("file path (dialog if empty)"="fmc", "format (%s)"="%s" ("format (%.3f)"), "delimiter (\\t)"="," ("delimiter (\\t)")) -> ("all rows"=w2:string[][])  [unwired: 7 in, 5 out]
  "all rows" <- w2
  n4 = Index Array(array=w20, index (col)=0 ("disabled index (col)")) -> (element=w19:string[])  [unwired: 1 in]
  "subarray" <- w19
  n5 = Index Array(array=w2, index (col)=1 ("disabled index (col)")) -> (element=w9:string[])  [unwired: 1 in]
  "subarray 2" <- w9
  n6 = Index Array(array=w2, index (col)=0 ("disabled index (col)")) -> (element=w1:string[])  [unwired: 1 in]
  n7 = for {
    N: 64 -> [_]
    tunnel: w19 -> [w29]
    shift-right: [w27] -> w5
    shift-left: w17 -> [w28]
    tunnel: w9 -> [w25] mode=indexing
    tunnel: w1 -> [w26] mode=indexing
    n8 = case shown="True" "-N" {
      tunnel: w25 -> [w30 w32]
      tunnel: [w30 w31] -> w24
      frame False {
      }
      frame True {
        n9 = Search and Replace String(input string=w32, search string="_P", replace string="_N" ("search string")) -> (result string=w31:string)  [unwired: 5 in, 3 out]
      }
    }
    n10 = for {
      tunnel: w29 -> [w56] mode=indexing
      tunnel: w29 -> [w53]
      shift-right: [w50] -> w27
      shift-left: w28 -> [w51]
      tunnel: w24 -> [w37]
      tunnel: w26 -> [w35]
      i -> [w52]
      n11 = Concatenate Strings("prefix", w37) -> (w38:string)
      n12 = Match Pattern(string=w56, regular expression=w38) -> (before substring=w44:string, after substring=w49:string, offset past match=w55:i32)  [unwired: 1 in, 1 out]
      n13 = Match Pattern(string=w44, regular expression="PACKAGE_PIN ") -> (after substring=w39:string, offset past match=w41:i32)  [unwired: 1 in, 2 out]
      n14 = Equal?(x="]", y=w49) -> (x = y?=w47:bool)
      n15 = Not Equal?(x=w55, y=-1) -> (x != y?=w46:bool)
      n16 = Not Equal?(x=-1 ("y"), y=w41) -> (x != y?=w40:bool)
      n17 = Compound Arithmetic op=AND(w40, w47, w46) -> (w45:bool)
      n18 = case shown="True" w45 {
        tunnel: w53 -> [_ _]
        tunnel: w52 -> [_ _]
        tunnel: [w57 w63] -> w50
        tunnel: w51 -> [w57 w62]
        tunnel: w38 -> [_ w61]
        tunnel: w39 -> [_ w60]
        tunnel: w35 -> [_ w58]
        frame False {
        }
        frame True {
          n19 = Match Pattern(string=w60, regular expression=" ") -> (before substring=w59:string, offset past match=w65:i32)  [unwired: 1 in, 2 out]
          n20 = Not Equal?(x=w65, y=-1) -> (x != y?=w64:bool)
          n21 = case shown="True" w64 {
            tunnel: [w68 w74] -> w63
            tunnel: w62 -> [w68 w73]
            tunnel: w61 -> [_ w72]
            tunnel: w59 -> [_ w71]
            tunnel: w58 -> [_ w69]
            frame False {
            }
            frame True {
              n22 = Build Array(w69, w72, w71) -> (w70:string[])
              n23 = Build Array (concatenate)(w73, w70) -> (w74:string[][])
            }
          }
        }
      }
    }
  }
  n24 = Array Subset(array=w5, index (row)=1 ("index")) -> (→"Array":string[][])  [unwired: 3 in]
